vi "Dashboard Main.vi"() -> ()   [LabVIEW 2019]
uses:
  <vilib>/Utility/miscctls.llb/LVRowAndColumnTypeDef.ctl
  <vilib>/event_ctls.llb/eventvkey.ctl
  <vilib>/Rock Robotics/Network Tables/NT Write Boolean.vi
  <vilib>/Utility/file.llb/Read Delimited Spreadsheet (string).vi
  <vilib>/Rock Robotics/Network Tables/NT Write String Array.vi
  <vilib>/Rock Robotics/WPI/Dashboard/WPI_DashboardLogging Global.vi
panel:
  in  "Camera Settings Right":T1={"Frame Rate"=30, "Compression"=30, "Size"=1, "DB Camera Config"=FALSE} {"Frame Rate" scale=1.0..30.0; "Compression" scale=100.0..-1.0; "Size" items=["640x480", "320x240", "160x120"]}
  in  "Camera Name Right":string(combo)="No Camera Selection"
  out "Camera Perf":string
  in  "Camera Settings":T1={"Frame Rate"=30, "Compression"=30, "Size"=1, "DB Camera Config"=FALSE} {"Frame Rate" scale=1.0..30.0; "Compression" scale=100.0..-1.0; "Size" items=["640x480", "320x240", "160x120"]}
  in  "TCP":refnum<k5>
  in  "Rec Mode":enum32{"Stop", "Record", "Playback"}(radio)
  out "Robot IP":string
  out "Image Message":string="Timeout in Camera Communications"
  in  "Dashboard Tab":T2(tab)
  in  "Select Auto":string(combo)="Select Autonomous ..."
  out "NT Connection":bool
  out "JS1 Z":dbl(slide) scale=-1.0..1.0 scale format="%#_2e"
  out "JS1 Graph":cluster{"X":dbl, "Y":dbl}[](graph)
  out "JS1 Buttons":T3
  out "JS2 Z":dbl(slide) scale=-1.0..1.0 scale format="%#_2e"
  out "JS2 Graph":cluster{"X":dbl, "Y":dbl}[](graph)
  out "JS2 Buttons":T3
  out "Mode":T4(ring)=enum."Auto Disabled"
  out "Right Camera Perf":cluster{"Bandwidth (Mbps)":dbl, "FPS":dbl}
  out "Camera Image Right":T5(plugin-control)
  in  "DB/String 9":string
  in  "DB/String 8":string
  in  "DB/String 7":string
  in  "DB/String 6":string
  in  "DB/String 5":string
  in  "DB/String 4":string
  in  "DB/String 3":string
  in  "DB/String 2":string
  in  "DB/String 1":string
  in  "DB/String 0":string
  in  "DB/Slider 0":dbl(slide) scale=0.0..5.0
  in  "DB/Slider 1":dbl(slide) scale=0.0..5.0
  in  "DB/Slider 2":dbl(slide) scale=0.0..5.0
  in  "DB/Slider 3":dbl(slide) scale=0.0..5.0
  out "DB/LED 3":bool
  out "DB/LED 2":bool
  out "DB/LED 1":bool
  out "DB/LED 0":bool
  in  "DB/Button 3":bool
  in  "DB/Button 2":bool
  in  "DB/Button 1":bool
  in  "DB/Button 0":bool caption="New Name"
  in  "Test Slider":dbl(slide) scale=0.0..100.0 scale format="%#_3g"
  in  "On/Off":bool caption="Solenoid"
  in  "Test Name":u16(ring) items=["Select the test to run..."]
  in  "Test Tree":string(tree)
  in  "Motor":cluster{"Value":dbl, "Enable":bool} {"Value" scale=-1.0..1.0 scale format="%#_3g"}
  out "Progress":T6 {"Test Progress" scale=0.0..100.0}
  in  "Rev/Fwd":cluster{"Forward":bool, "Reverse":bool}
  in  "Test Ring":u16(ring) items=["Monochrome", "Color"]
  out "Cmd Status":string
  in  "Execute Command":bool
  in  "Command Params":string[][](table)
  in  "Command Selection":i32(listbox)
  in  "CheckList":i32(listbox)
  out "Tree":string(tree)
  out "Magazine":enum32{"Controls", "Indicators"}(tab)
  in  "Max Magazine Speed":dbl
  in  "Unjam Speed":dbl
  in  "Firing Speed":dbl
  in  "Loading Speed":dbl
  in  "Bottom IR Theshold":dbl
  in  "Bottom Middle IR Threshold":dbl
  in  "Top Middle IR Threshold":dbl
  in  "Top IR Threshold":dbl
  out "Current Max Magazine Speed":dbl
  out "Current Unjam Speed":dbl
  out "Current Firing Speed":dbl
  out "Current Loading Speed":dbl
  out "Current Bottom IR Threshold":dbl
  out "Current Bottom Middle IR Threshold":dbl
  out "Current Top Middle IR Threshold":dbl
  out "Current Top IR Threshold":dbl
  in  "Boolean":bool
  out "Drive":enum32{"Controls", "Indicators"}(tab)
  in  "Left P":dbl
  in  "Left I":dbl
  in  "Left D":dbl
  in  "Left F":dbl
  in  "Right P":dbl
  in  "Right I":dbl
  in  "Right D":dbl
  in  "Right F":dbl
  out "Current Right F":dbl
  out "Current Right D":dbl
  out "Current Right I":dbl
  out "Current Right P":dbl
  out "Current Left F":dbl
  out "Current Left D":dbl
  out "Current Left I":dbl
  out "Current Left P":dbl
  out "Flywheel":enum32{"Controls", "Indicators"}(tab)
  in  "Flywheel Max":dbl
  in  "Flywheel Min":dbl
  in  "Flywheel I":dbl
  in  "Flywheel F":dbl
  in  "Flywheel D":dbl
  in  "Flywheel I":dbl
  in  "Flywheel P":dbl
  out "Current Flywheel Max":dbl
  out "Current Flywheel Min":dbl
  out "Current Flywheel I":dbl
  out "Current Flywheel F":dbl
  out "Current Flywheel D":dbl
  out "Current Flywheel I":dbl
  out "Current Flywheel P":dbl
  out "Turret":enum32{"Controls", "Indicators"}(tab)
  in  "Turret Upper Limit":dbl
  in  "Turret Lower Limit":dbl
  out "Current Turret Lower Limit":dbl
  out "Current Turret Upper Limit":dbl
  out "Climb":enum32{"Controls", "Indicators"}(tab)
  in  "Climb I":dbl
  in  "Climb P":dbl
  in  "Climb D":dbl
  out "Current Climb D":dbl
  out "Current Climb I":dbl
  out "Current Climb P":dbl
  out "Intake":enum32{"Controls", "Indicators"}(tab)
  in  "extend delay(ms)":dbl
  in  "retract delay(ms)":dbl
  in  "Intake Speed":dbl
  out "Current Intake Speed":dbl
  out "Current Magazine Speed":dbl
  out "Match Color":string
  in  "Auto Selector":u16(ring) items=["Trench Play", "Move Off Line", "No Auto"]
  out "Camera Image":T5(plugin-control)
  out "Background":bool
  in  "Camera Name":string(combo)="No Camera Selection"
  # "HW"
  # "HW"
  # "Joysticks"
  # "Drive Motors"
  # "Front"
  # "Right"
  # "Left"
  # "Back"
  # "This tab is a great place for autonomous settings and robot-specific values.\nPlace controls and indicators inside this tab and match name to\nDashboard Variables on robot. You can also delete this comment."
  # "Read"
  # "Write"
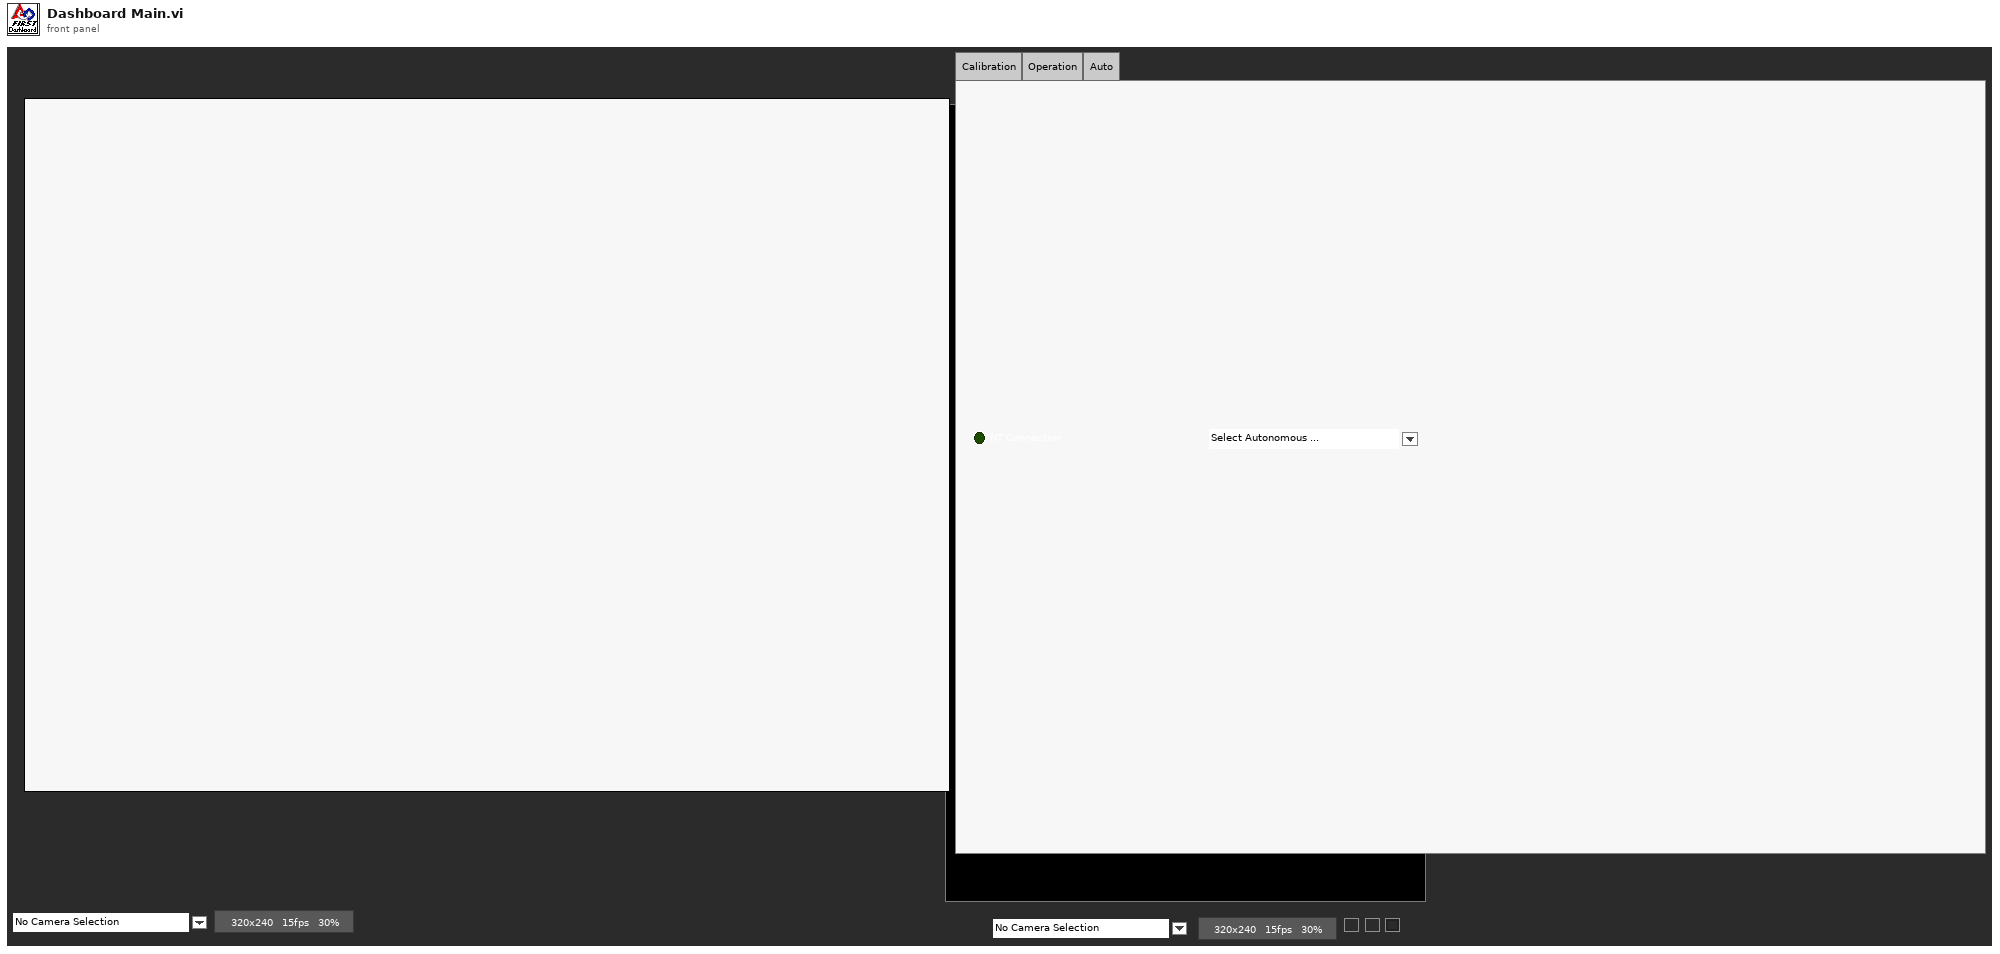
[diagram p1: front panel]
types:
  T1 = cluster{"Frame Rate":i32, "Compression":i32, "Size":u16, "DB Camera Config":bool}
  T2 = enum32{"Drive", "Camera", "Basic", "Custom", "Test", "Commands", "Checklist", "Variables", "Calibration", "Operation", "Auto"}
  T3 = cluster{bool, bool, bool, bool, bool, bool, bool, bool, bool, bool, bool, bool}
  T4 = enum8{"Tele-Op Disabled", "Tele-Op Enabled", "Auto Disabled", "Auto Enabled", "Test Disabled", "Test Enabled", "Disconnected", "No Code", "E-Stop"}
  T5 = typedef "IMAQ Image.ctl" = refnum<image>
  T6 = cluster{"Test Progress":u8, "Test Progress Text":string}
  T7 = cluster{"Save Path":path, "Interval (s)":dbl, "Keep":i32}
  T8 = enum32{"Drive", "Camera", "Basic", "Custom", "Test", "Commands", "Checklist", "Variables"}
  T9 = typedef "Image Type" = u32
  T10 = cluster{"IDs":cluster{"RPC field ID":u16, "Unique ID":u16}, "String":string}
  T11 = cluster{"Error Strings":string, "Disable Counts":cluster{u16, u16}, "Rail Faults":cluster{u16, u16, u16}, "Robot IP":string, "DB Mode":u8, "Event Info":cluster{"Name":string, "Type":u8, "Number":u16, "Replay":u8}}
  T12 = cluster{"Storage":cluster{"Disk Free":u64, "RAM Block":u32, "RAM free":u32}, "CPU Utilization":cluster{"CPU % ISR":sgl, "CPU % Time Crit":sgl, "CPU % Timed Str":sgl, "CPU % High":sgl, "CPU % Above":sgl, "CPU % Normal":sgl, "CPU % Low":sgl}, "CAN":cluster{"% Bus Utilization":sgl, "Bus Off Cnt":u32, "TX_FIFO Full Cnt":u32, "Receive Error Cnt":u8, "Transmit Error Cnt":u8}, "HID":cluster{"HID Outputs":u32, "Rumble Low":u16, "Rumble High":u16}[]}
  T13 = cluster{"Status bits":cluster{"Test Mode":bool, "Autonomous":bool, "Enabled":bool, "Code Start":bool, "Brownout":bool, "Reserved 2":bool, "Reserved 3":bool, "E-Stop":bool}, "Code Trace":cluster{"Disabled":bool, "TeleOp":bool, "Auto":bool, "Test":bool}, "Controller Type":enum16{"unknown", "cRIO", "roboRio"}, "Code?":enum16{"unknown", "noCode", "code"}, "Battery V":dbl}
  T14 = cluster{"Control Bits":cluster{"TestMode":bool, "Autonomous":bool, "Enabled":bool, "FMS Present":bool, bool, bool, bool, "E-Stop":bool}, "Team Station ":u8, "Countdown":sgl, "Joystick Values":cluster{"Axes":dbl[], "Buttons":bool[], "POVs":i16[]}[]}
  T15 = cluster{"Axes":dbl[], "Buttons":bool[], "POVs":i16[]}[]
  T16 = cluster{"Axes":dbl[], "Buttons":bool[], "POVs":i16[]}
  T17 = cluster{"Buttons[0]":bool, "Buttons[1]":bool, "Buttons[2]":bool, "Buttons[3]":bool, "Buttons[4]":bool, "Buttons[5]":bool, "Buttons[6]":bool, "Buttons[7]":bool, "Buttons[8]":bool, "Buttons[9]":bool, "Buttons[10]":bool, "Buttons[11]":bool}
  T18 = cluster{"Camera Image":refnum<vi>, "Dashboard Tab":refnum<vi>, "Background":refnum<vi>, "Rec Mode":refnum<vi>, "Test Slider":refnum<vi>, "On/Off ":refnum<vi>, "Test Ring":refnum<vi>, "Rev/Fwd":refnum<vi>, "Test Name":refnum<vi>, "Motor":refnum<vi>, "Progress":refnum<vi>, "CheckList":refnum<vi>, "Tree":refnum<vi>, "Test Tree":refnum<vi>, "Command Params":refnum<vi>, "Command Selection":refnum<vi>, "Execute Command":refnum<vi>, "Cmd Status":refnum<vi>, "Camera Settings":refnum<vi>, "Camera Name":refnum<vi>, "Camera Perf":refnum<vi>, "Camera Settings Right":refnum<vi>, "Camera Name Right":refnum<vi>, "Camera Image Right":refnum<vi>}
  T19 = cluster{"Global Rectangle":i32[], "Contours":cluster{"Contour Type":u32, "ROI Type":u32, "Points":i32[]}[]}
  T20 = cluster{"Camera Name":string, string, "Saved DB Images Info":cluster{"Save Path":path, "Interval (s)":dbl, "Keep":i32}}
  T21 = cluster{"Camera Name Right":string, string, "Saved DB Images Info":cluster{"Save Path":path, "Interval (s)":dbl, "Keep":i32}}
  T22 = cluster{"Operation":enum16{"Update", "Clear"}, "Color Box":u32}[]
  T23 = typedef "eventvkey.ctl" = enum16{"ASCII", "Enter", "Return", "Shift", "Ctrl", "Alt", "Cmd", "Opt", "Caps", "NumLock", "Clear", "Break", "Up", "Down", "Left", "Right", "Insert", "Delete", "Home", "End", "PageUp", "PageDown", "Escape", "Help", "Pause", "ScrollLock", "F1", "F2", "F3", "F4", "F5", "F6", "F7", "F8", "F9", "F10", "F11", "F12", "F13", "F14", "F15", "F16", "F17", "F18", "F19", "F20", "F21", "F22", "F23", "F24", "Play", "VolumeUp", "VolumeDown", "Mute", "Two Byte Char"}
  T24 = cluster{"Image Size":bool, "Image Type":bool, "Pixel Value":bool, "ROI Information":bool, "Zoom Factor":bool}
  T25 = cluster{"Operation":enum16{"Update", "Clear"}, "Color Box":u32}
  T26 = typedef "LVRowAndColumnTypeDef.ctl" = cluster{"Row":i32, "Column":i32}
  T27 = cluster{"Shift":bool, "Ctrl":bool, "Alt":bool, "Cmd":bool, "Opt":bool}
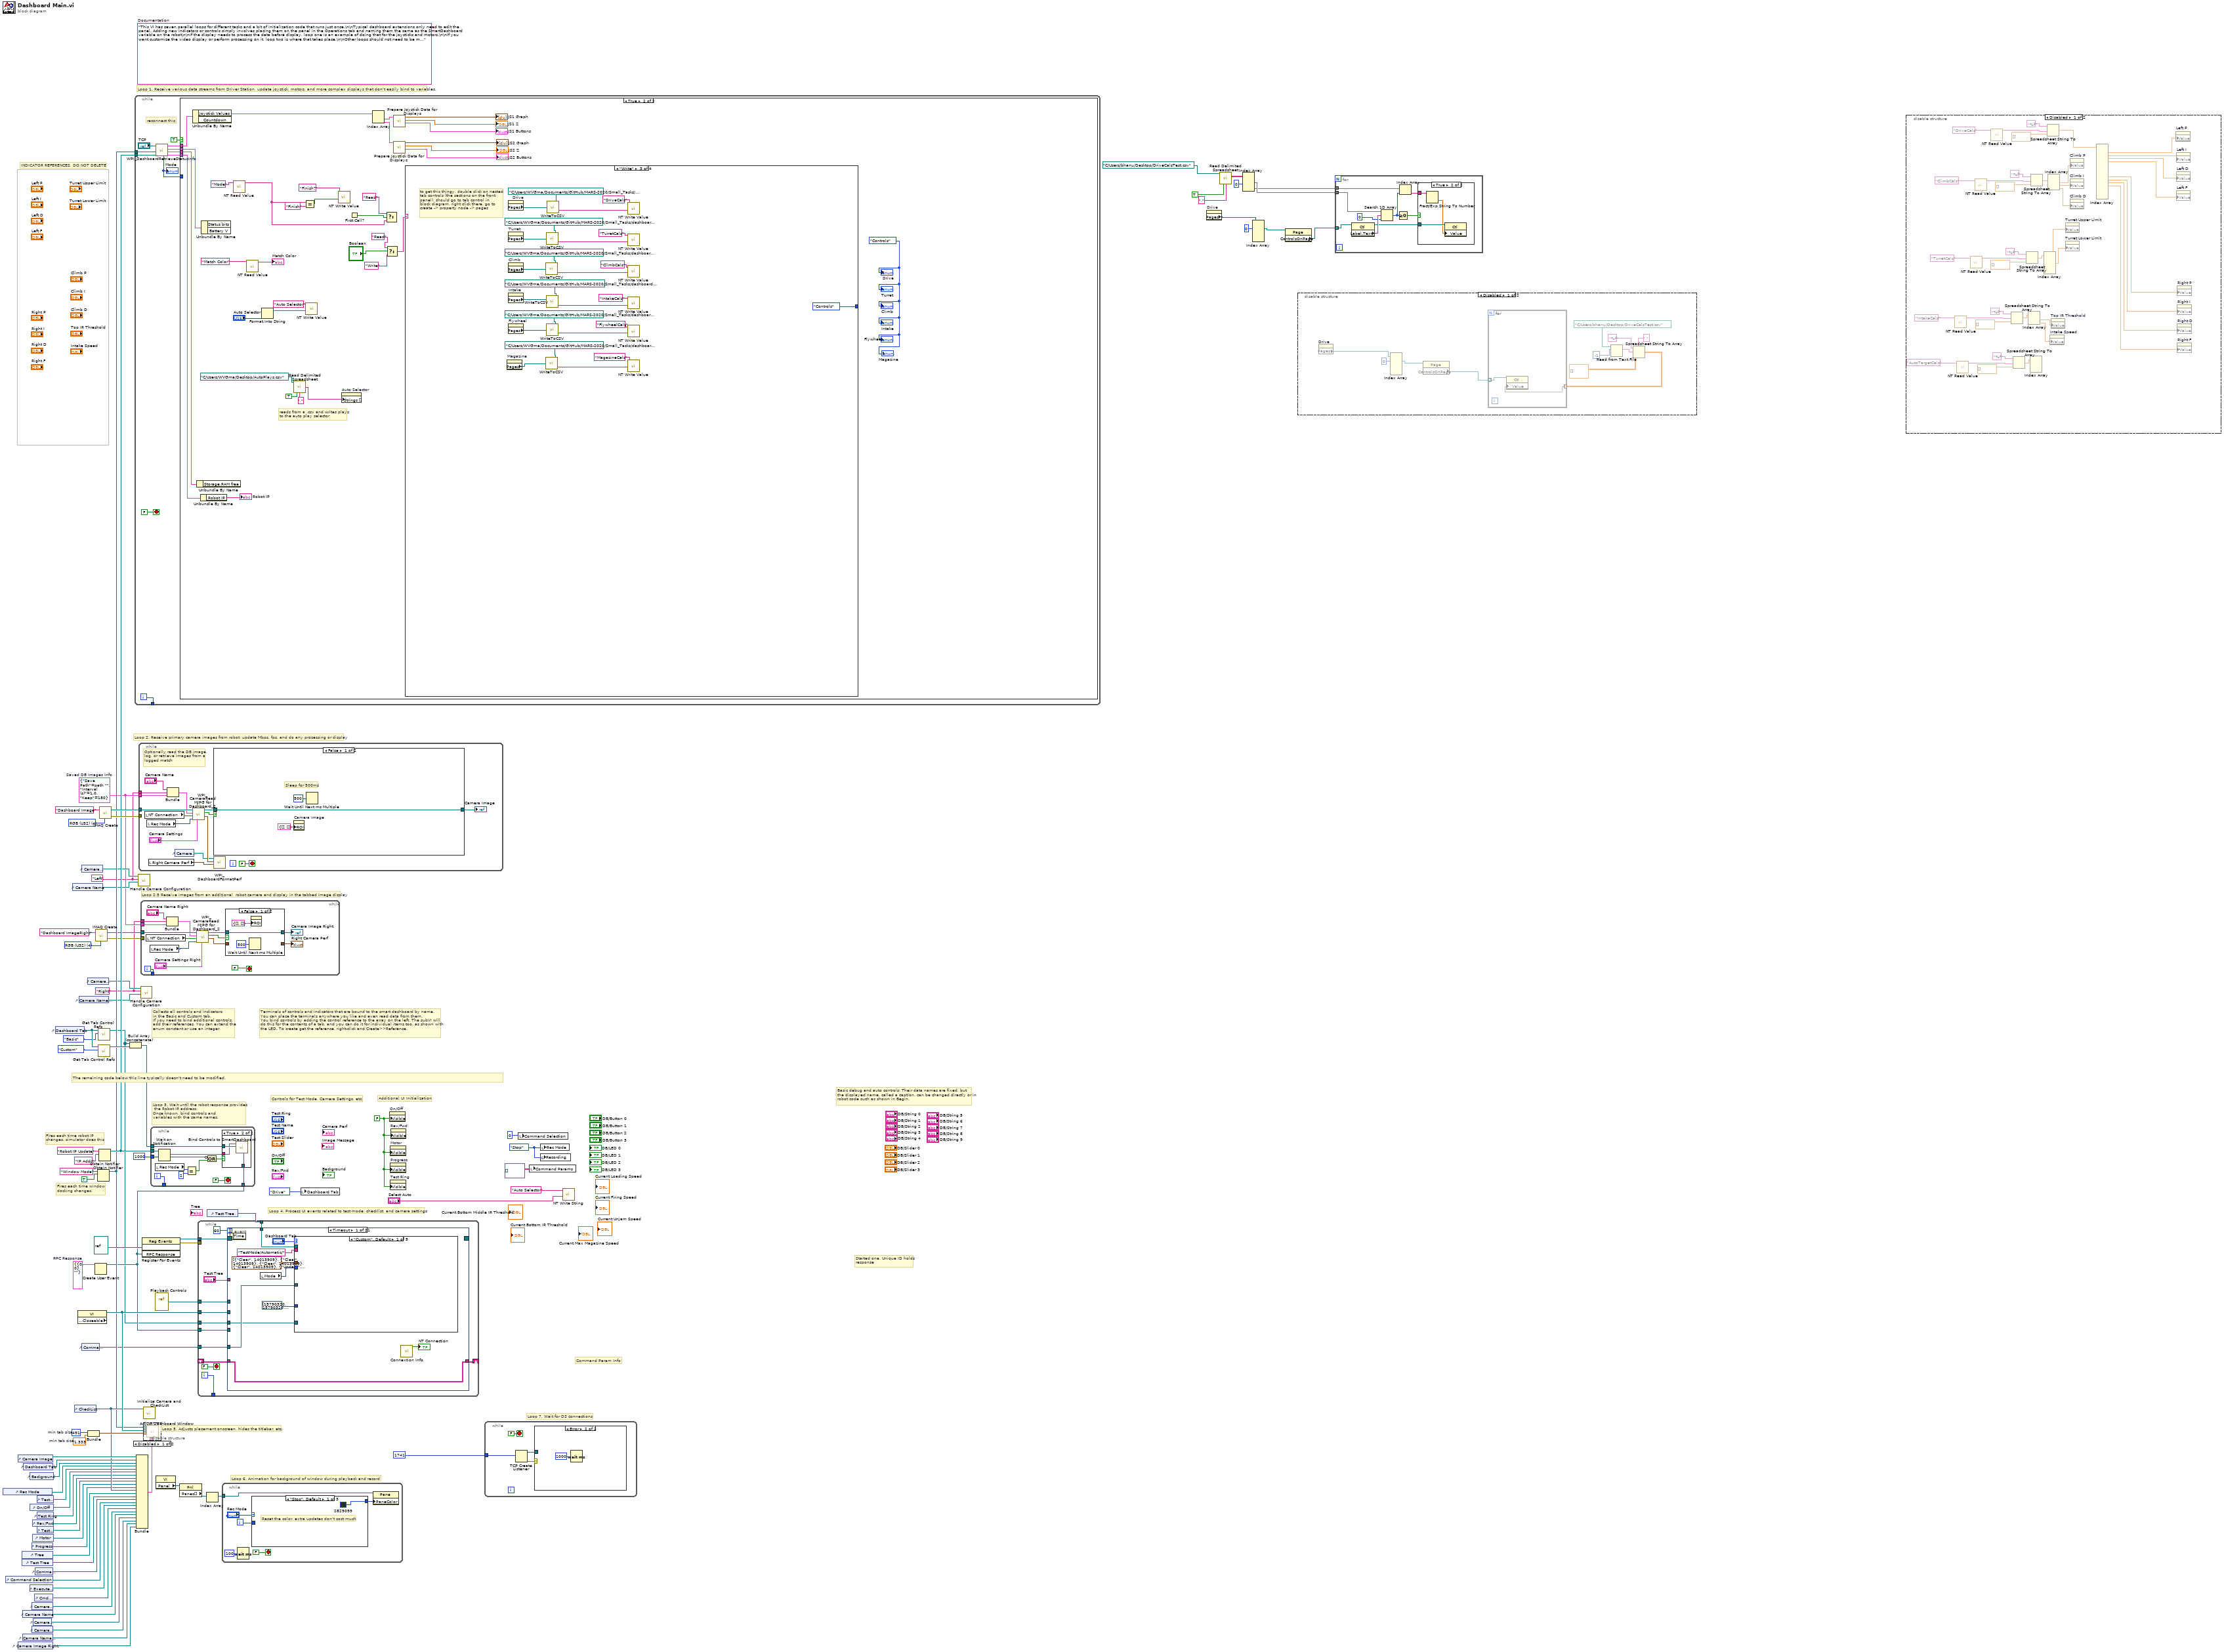
[diagram p0: block diagram]
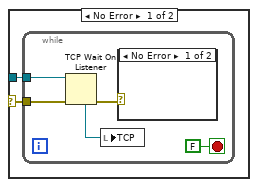
[diagram p7: hidden frame]
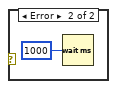
[diagram p8: hidden frame]
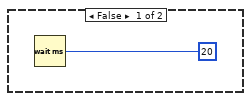
[diagram p9: hidden frame]
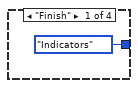
[diagram p10: hidden frame]
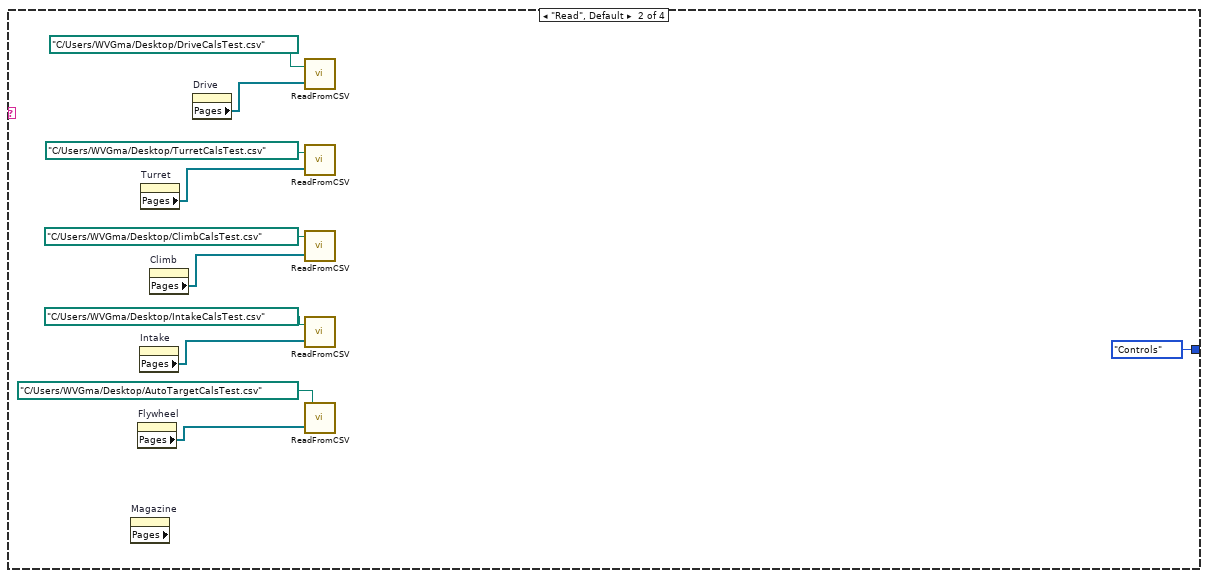
[diagram p11: hidden frame]
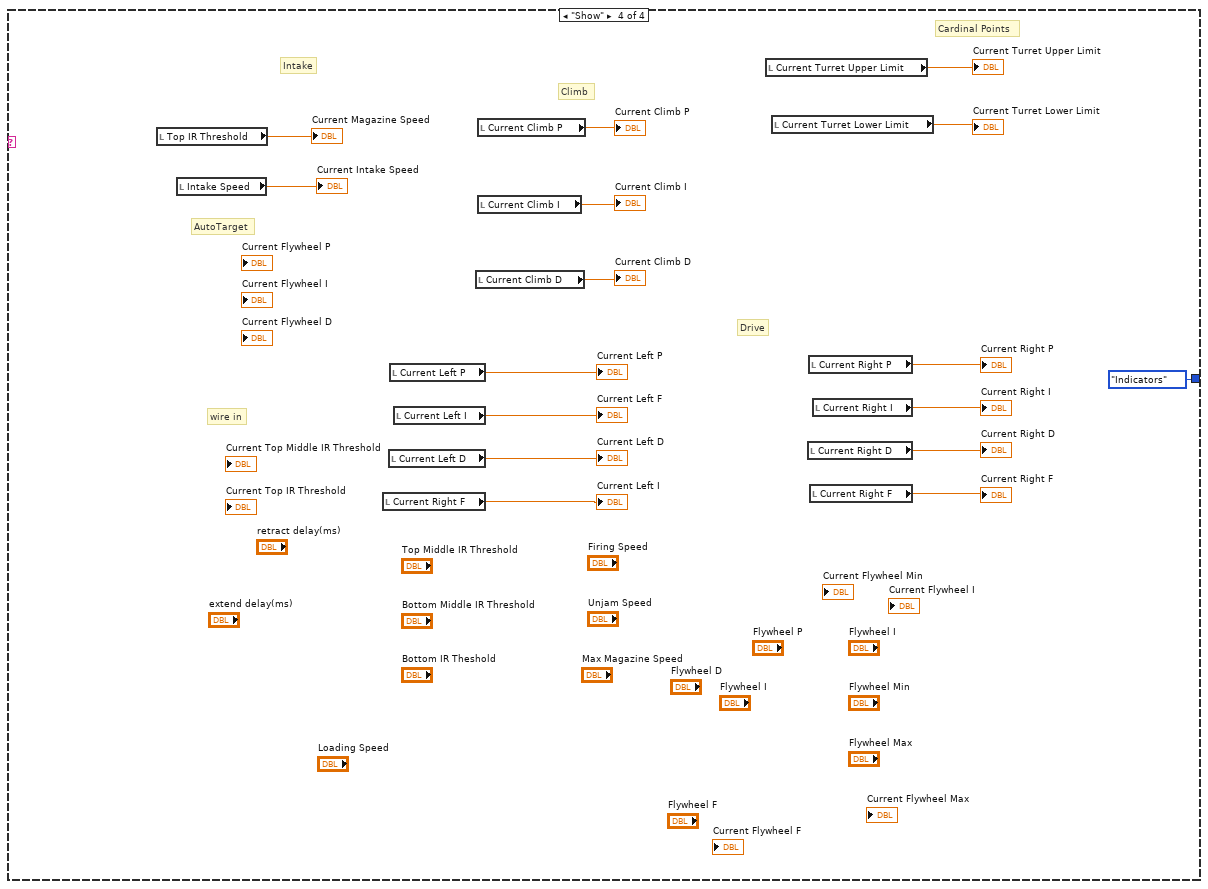
[diagram p12: hidden frame]
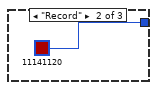
[diagram p13: hidden frame]
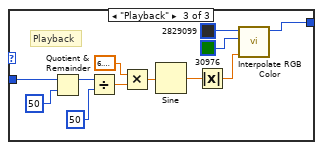
[diagram p14: hidden frame]
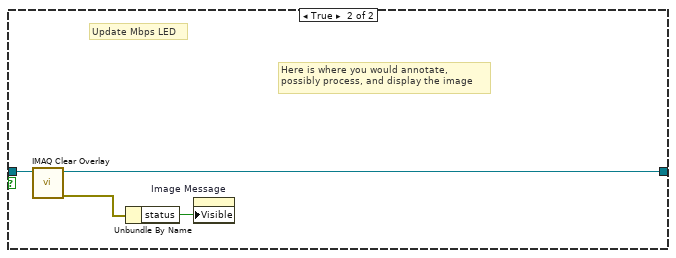
[diagram p16: hidden frame]
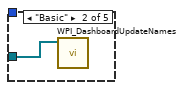
[diagram p17: hidden frame]
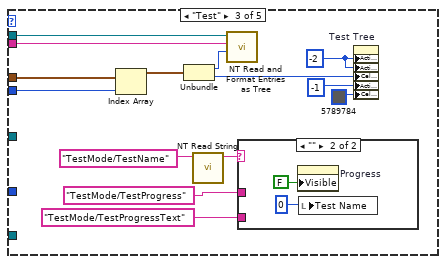
[diagram p18: hidden frame]
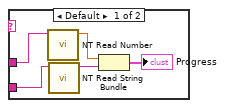
[diagram p19: hidden frame]
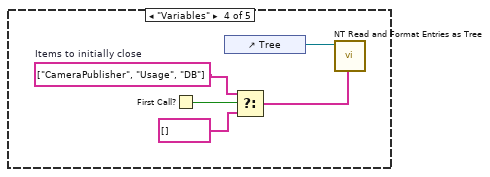
[diagram p20: hidden frame]
diagram:
  w14 = T7 {"Save Path"=path "", "Interval (s)"=1.0, "Keep"=180}  # Saved DB Images Info
  w13 = "Right"
  w12 = "Left"
  w24 = T9 4 items=["Grayscale (U8)", "Grayscale (I16)", "Grayscale (SGL)", "Complex (CSG)", "RGB (U32)", "HSL (U32)", "RGB (U64)"] ("Image Type")
  w40 = T10 {"IDs"={"RPC field ID"=0, "Unique ID"=0}, "String"=""}  # RPC Response
  w63 = 491  # min tab size
  w62 = 1.333  # min tab size
  w70 = enum32{"Stop", "Record", "Playback"}."Stop" ("Rec Mode")
  w47 = FALSE ("Visible")
  (unwired) "This VI has seven parallel loops for different tasks and a bit of initialization code that runs just once.\n\nTypical dashboard extensions only need to edit the panel. Adding new indicators or controls simply involves placing them on the panel in the Operations tab and naming them the same as the SmartDashboard variable on the robot\n\nIf the display needs to process the data before display, loop one is an example of doing that for the joysticks and motors.\n\nIf you want customize the video display or perform processing on it, loop two is where that takes place.\n\nOther loops should not need to be modified. They are pretty standard, and document the task they perform."  # Documentation
  w87 = T9 4 items=["Grayscale (U8)", "Grayscale (I16)", "Grayscale (SGL)", "Complex (CSG)", "RGB (U32)", "HSL (U32)", "RGB (U64)"] ("Image Type")
  # "INDICATOR REFERENCES, DO NOT DELETE"
  # "Loop 2.5 Receive images from an additional  robot camera and display in the tabbed image display"
  # "Command Param Info"
  # "Started one, Unique ID holds\nresponse"
  # "Loop 7. Wait for DS connections"
  # "Basic debug and auto controls: Their data names are fixed, but\nthe displayed name, called a caption, can be changed directly or in\nrobot code such as shown in Begin."
  # "Controls for Test Mode, Camera Settings, etc."
  # "Additional UI Initialization"
  # "Loop 6. Animation for background of window during playback and record"
  # "Fires each time robot IP\nchanges, simulator does this"
  # "Fires each time window\ndocking changes."
  # "Collects all controls and indicators\nin the Basic and Custom tab.\nIf you need to bind additional controls,\nadd their references. You can extend the\nenum constant or use an integer."
  # "The remaining code below this line typically doesn't need to be modified."
  # "Loop 4. Process UI events related to test mode, checklist, and camera settings"
  # "Terminals of controls and indicators that are bound to the smart dashboard by name.\nYou can place the terminals anywhere you like and even read data from them.\nYou bind controls by adding the control reference to the array on the left. The subVI will\ndo this for the contents of a tab, and you can do it for individual items too, as shown with\nthe LED. To create get the reference, right-click and Create>>Reference."
  # "Loop 3. Wait until the robot response provides\n the Robot IP address.\nOnce known, bind controls and\nvariables with the same names."
  # "Loop 5. Adjusts placement onscreen, hides the titlebar, etc."
  # "Loop 1. Receive various data streams from Driver Station, update joystick, motors, and more complex displays that don't easily bind to variables."
  # "Loop 2. Receive primary camera images from robot, update Mbps, fps, and do any processing or display"
  n1 = control-ref of="Rec Mode"() -> (w53:refnum<vi>)
  n2 = control-ref of="Command Selection"() -> (w39:refnum<vi>)
  n3 = control-ref of="Camera Image Right"() -> (w17:refnum<vi>)
  n4 = control-ref of="Camera Image"() -> (w65:refnum<vi>)
  n5 = control-ref of="Tree"() -> (w57:refnum<vi>)
  n6 = control-ref of="Test Tree"() -> (w56:refnum<vi>)
  n7 = control-ref of="Camera Name"() -> (w30:refnum<vi>)
  n8 = control-ref of="Camera Name Right"() -> (w18:refnum<vi>)
  n9 = control-ref of="Dashboard Tab"() -> (w64:refnum<vi>)
  n10 = control-ref of="Execute Command"() -> (w41:refnum<vi>)
  n11 = control-ref of="Background"() -> (w60:refnum<vi>)
  n12 = control-ref of="On/Off"() -> (w51:refnum<vi>)
  n13 = control-ref of="Progress"() -> (w48:refnum<vi>)
  n14 = control-ref of="Camera Settings"() -> (w31:refnum<vi>)
  n15 = control-ref of="Camera Settings Right"() -> (w19:refnum<vi>)
  n16 = control-ref of="Rev/Fwd"() -> (w49:refnum<vi>)
  n17 = control-ref of="Motor"() -> (w54:refnum<vi>)
  n18 = control-ref of="Camera Perf"() -> (w29:refnum<vi>)
  n19 = control-ref of="Cmd Status"() -> (w35:refnum<vi>)
  n20 = control-ref of="Command Params"() -> (w42:refnum<vi>)
  n21 = control-ref of="Test Slider"() -> (w52:refnum<vi>)
  n22 = control-ref of="Test Ring"() -> (w50:refnum<vi>)
  n23 = control-ref of="Test Name"() -> (w55:refnum<vi>)
  n24 = control-ref of="Dashboard Tab"() -> (w68:refnum<vi>)
  n25 = control-ref of="Camera Name"() -> (w32:refnum<vi>)
  n26 = control-ref of="CheckList"() -> (w58:refnum<vi>)
  n27 = property class="VI" props=["Front Panel.Closeable"]() -> (reference out=w69:refnum<vi>)  [unwired: 2 in, 2 out]
  n28 = control-ref of="Camera Name Right"() -> (w20:refnum<vi>)
  n29 = control-ref of="Camera Settings"() -> (w33:refnum<vi>)
  n30 = control-ref of="Command Params"() -> (w34:refnum<vi>)
  n31 = control-ref of="Camera Settings Right"() -> (w21:refnum<vi>)
  n32 = Bundle("min tab size"=w63, "min tab size"=w62) -> (w61:cluster{"min tab size":i32, "min tab size":dbl})  [unwired: 1 in]
  n33 = Create User Event(user event datatype=w40) -> (user event=w36:refnum<user-event>)  [unwired: 1 in, 1 out]
  n34 = call "IMAQ Create"("Image Name"="Dashboard ImageRight", "Image Type"=w24) -> ("New Image"=w23:T5, "error out"=w22:errorcluster)  [unwired: 2 in, 1 out]
  n35 = Obtain Notifier(name (unnamed)="Window Mode", notification data type=TRUE) -> (notifier out=w45:refnum<notifier>)  [unwired: 2 in, 2 out]
  n36 = call <vilib>:"Get Tab Control Refs.vi"("Page Index"=T8."Basic" ("Dashboard Tab"), "TabControl in"=w68) -> ("ControlsOnPage"=w28:refnum<vi>[])  [unwired: 9 in]
  n37 = call <vilib>:"Get Tab Control Refs.vi"("Page Index"=T8."Custom" ("Dashboard Tab"), "TabControl in"=w68) -> ("ControlsOnPage"=w67:refnum<vi>[])  [unwired: 9 in]
  n38 = Obtain Notifier(name (unnamed)="Robot IP Update", notification data type="IP Addr" ("name (unnamed)")) -> (notifier out=w46:refnum<notifier>)  [unwired: 2 in, 2 out]
  n39 = call "IMAQ Create"("Image Name"="Dashboard Image", "Image Type"=w87) -> ("New Image"=w85:T5, "error out"=w84:errorcluster)  [unwired: 2 in, 1 out]
  n40 = Build Array (concatenate)(w28, w67) -> (w66:refnum<vi>[])
  n41 = while {
    tunnel: [w97] -> _
    tunnel: w46 -> [w92]
    tunnel: w45 -> [w89]
    i -> [w97]
    stop <- FALSE stop-if-true
    # "reconnect this"
    n42 = call <vilib>:"WPI_DashboardRetrieveStatusInfo.vi"("Binding Refnum"=w92, "Window Mode Notifier"=w89, "TCP Cnx"="TCP") -> ("Power and Errors"=w93:T11, "Robot Metrics"=w95:T12, "Status Info"=w96:T13, "Control Info"=w94:T14, "Robot Mode"=w91:T4)  [unwired: 3 in, 1 out]
    "Mode" <- w91
    n43 = case shown="True" TRUE {
      tunnel: w96 -> [_ w134]
      tunnel: w95 -> [_ w133]
      tunnel: w94 -> [_ w132]
      tunnel: w93 -> [_ w131]
      tunnel: w91 -> [_ _]
      frame False {
        n44 = Wait (ms)(milliseconds to wait=u32 20) -> ()  [unwired: 1 out]
      }
      frame True {
        w100 = enum32{"Controls", "Indicators"}."Controls" ("Climb")
        # "reads from a .csv and writes plays\nto the auto play selector"
        n45 = Unbundle By Name(w132) -> ("Joystick Values"=w130:T15)  [unwired: 1 out]
        n46 = Unbundle By Name(w133) -> ()  [unwired: 1 out]
        n47 = Unbundle By Name(w131) -> ("Robot IP"=→"Robot IP":string)
        n48 = Unbundle By Name(w134) -> ()  [unwired: 2 out]
        n49 = call-poly <vilib>:"NT Read Value.vi"("Name"="Mode") -> ("String"=w114:string)  [unwired: 9 in, 1 out]
        n50 = call-poly <vilib>:"NT Read Value.vi"("Name"="Match Color") -> ("String"=→"Match Color":string)  [unwired: 9 in, 1 out]
        n51 = Format Into String("Auto Selector") -> (resulting string=w111:string)  [unwired: 3 in, 1 out]
        n52 = call-poly <vilib>:"Read Delimited Spreadsheet.vi"("file path (dialog if empty)"=path "C:/Users/WVGma/Desktop/AutoPlays.csv", "transpose? (F)"=TRUE, "delimiter (\\t)"="," ("delimiter (\\t)")) -> ("first row"=w105:string[])  [unwired: 7 in, 5 out]
        n53 = Equal?(x=w114, y="Finish") -> (x = y?=w118:bool)
        n54 = call-poly <vilib>:"NT Write Value.vi"("String"=w111, "Name"="Auto Selector") -> ()  [unwired: 9 in, 1 out]
        n55 = call-poly <vilib>:"NT Write Value.vi"("Boolean"=w118, "Name"="Finish?") -> ()  [unwired: 9 in, 1 out]
        n56 = property on="Auto Selector" class="Ring (strict)"("Strings []"=w105) -> ()  [unwired: 2 in, 2 out]
        n57 = First Call?() -> (First Call?: T/F=w116:bool)
        n58 = Index Array(array=w130) -> (element #1=w129:T16, element #2=w125:T16)  [unwired: 2 in]
        n59 = Select(t="Read" ("f"), s=w116, f=w114) -> ()  [unwired: 1 out]
        n60 = Select(t="Read", s="Boolean", f="Write") -> (s? t:f=w101:string)
        n61 = call "Prepare Joystick Data for Displays.vi"("Joystick Values"=w125) -> ("Buttons"=→"JS2 Buttons":T17, "Z Axis"=→"JS2 Z":dbl, "Cartesian Data"=→"JS2 Graph":cluster{"X axis":dbl, "X axis":dbl}[])  [unwired: 8 in]
        n62 = call "Prepare Joystick Data for Displays.vi"("Joystick Values"=w129) -> ("Buttons"=→"JS1 Buttons":T17, "Z Axis"=→"JS1 Z":dbl, "Cartesian Data"=→"JS1 Graph":cluster{"X axis":dbl, "X axis":dbl}[])  [unwired: 8 in]
        n63 = case shown="\"Write\"" w101 {
          tunnel: [enum32{"Controls", "Indicators"}."Indicators" ("Climb") enum32{"Controls", "Indicators"}."Controls" ("Climb") enum32{"Controls", "Indicators"}."Controls" ("Climb") enum32{"Controls", "Indicators"}."Indicators" ("Climb")] -> _
          frame "Finish" {
          }
          frame "Read", Default {
            n64 = property on="Magazine" class="TabCtl (strict)" props=["Pages"]() -> ()  [unwired: 2 in, 3 out]
            n65 = property on="Flywheel" class="TabCtl (strict)"() -> ("Pages"=w136:refnum<vi>[])  [unwired: 2 in, 2 out]
            n66 = property on="Intake" class="TabCtl (strict)"() -> ("Pages"=w137:refnum<vi>[])  [unwired: 2 in, 2 out]
            n67 = property on="Turret" class="TabCtl (strict)"() -> ("Pages"=w142:refnum<vi>[])  [unwired: 2 in, 2 out]
            n68 = property on="Climb" class="TabCtl (strict)"() -> ("Pages"=w138:refnum<vi>[])  [unwired: 2 in, 2 out]
            n69 = property on="Drive" class="TabCtl (strict)"() -> ("Pages"=w144:refnum<vi>[])  [unwired: 2 in, 2 out]
            n70 = call "ReadFromCSV.vi"("Pages"=w144, "file path (dialog if empty)"=path "C:/Users/WVGma/Desktop/DriveCalsTest.csv") -> ()  [unwired: 1 in]
            n71 = call "ReadFromCSV.vi"("Pages"=w142, "file path (dialog if empty)"=path "C:/Users/WVGma/Desktop/TurretCalsTest.csv") -> ()  [unwired: 1 in]
            n72 = call "ReadFromCSV.vi"("Pages"=w138, "file path (dialog if empty)"=path "C:/Users/WVGma/Desktop/ClimbCalsTest.csv") -> ()  [unwired: 1 in]
            n73 = call "ReadFromCSV.vi"("Pages"=w137, "file path (dialog if empty)"=path "C:/Users/WVGma/Desktop/IntakeCalsTest.csv") -> ()  [unwired: 1 in]
            n74 = call "ReadFromCSV.vi"("Pages"=w136, "file path (dialog if empty)"=path "C:/Users/WVGma/Desktop/AutoTargetCalsTest.csv") -> ()  [unwired: 1 in]
          }
          frame "Write" {
            # "to get this thingy, double click on nested\ntab controls (the sections on the front \npanel), should go to tab control in \nblock diagram, right click there, go to\ncreate -> property node -> pages"
            n75 = property on="Magazine" class="TabCtl (strict)"() -> ("Pages"=w160:refnum<vi>[])  [unwired: 2 in, 2 out]
            n76 = property on="Drive" class="TabCtl (strict)"() -> ("Pages"=w161:refnum<vi>[])  [unwired: 2 in, 2 out]
            n77 = property on="Turret" class="TabCtl (strict)"() -> ("Pages"=w168:refnum<vi>[])  [unwired: 2 in, 2 out]
            n78 = property on="Climb" class="TabCtl (strict)"() -> ("Pages"=w169:refnum<vi>[])  [unwired: 2 in, 2 out]
            n79 = property on="Intake" class="TabCtl (strict)"() -> ("Pages"=w170:refnum<vi>[])  [unwired: 2 in, 2 out]
            n80 = property on="Flywheel" class="TabCtl (strict)"() -> ("Pages"=w167:refnum<vi>[])  [unwired: 2 in, 2 out]
            n81 = call "WriteToCSV.vi"("Pages"=w169, "file path (dialog if empty)"=path "C:/Users/WVGma/Documents/GitHub/MARS-2020/Small_Tasks/dashboard mOS XIII/Calibration Files/ClimbCals.csv") -> ("output array for NT"=w152:string[])
            n82 = call "WriteToCSV.vi"("Pages"=w160, "file path (dialog if empty)"=path "C:/Users/WVGma/Documents/GitHub/MARS-2020/Small_Tasks/dashboard mOS XIII/Calibration Files/MagazineCals.csv") -> ("output array for NT"=w154:string[])
            n83 = call "WriteToCSV.vi"("Pages"=w168, "file path (dialog if empty)"=path "C:/Users/WVGma/Documents/GitHub/MARS-2020/Small_Tasks/dashboard mOS XIII/Calibration Files/TurretCals.csv") -> ("output array for NT"=w157:string[])
            n84 = call "WriteToCSV.vi"("Pages"=w167, "file path (dialog if empty)"=path "C:/Users/WVGma/Documents/GitHub/MARS-2020/Small_Tasks/dashboard mOS XIII/Calibration Files/FlywheelCals.csv") -> ("output array for NT"=w155:string[])
            n85 = call "WriteToCSV.vi"("Pages"=w170, "file path (dialog if empty)"=path "C:/Users/WVGma/Documents/GitHub/MARS-2020/Small_Tasks/dashboard mOS XIII/Calibration Files/IntakeCals.csv") -> ("output array for NT"=w156:string[])
            n86 = call "WriteToCSV.vi"("Pages"=w161, "file path (dialog if empty)"=path "C:/Users/WVGma/Documents/GitHub/MARS-2020/Small_Tasks/dashboard mOS XIII/Calibration Files/DriveCals.csv") -> ("output array for NT"=w158:string[])
            n87 = call-poly <vilib>:"NT Write Value.vi"("String Array"=w158, "Name"="DriveCals") -> ()  [unwired: 9 in, 1 out]
            n88 = call-poly <vilib>:"NT Write Value.vi"("String Array"=w157, "Name"="TurretCals") -> ()  [unwired: 9 in, 1 out]
            n89 = call-poly <vilib>:"NT Write Value.vi"("String Array"=w152, "Name"="ClimbCals") -> ()  [unwired: 9 in, 1 out]
            n90 = call-poly <vilib>:"NT Write Value.vi"("String Array"=w156, "Name"="IntakeCals") -> ()  [unwired: 9 in, 1 out]
            n91 = call-poly <vilib>:"NT Write Value.vi"("String Array"=w155, "Name"="FlywheelCals") -> ()  [unwired: 9 in, 1 out]
            n92 = call-poly <vilib>:"NT Write Value.vi"("String Array"=w154, "Name"="MagazineCals") -> ()  [unwired: 9 in, 1 out]
          }
          frame "Show" {
            # "wire in"
            # "AutoTarget"
            # "Intake"
            # "Climb"
            # "Cardinal Points"
            # "Drive"
            n93 = local read "Top IR Threshold"() -> (→"Current Magazine Speed":dbl)
            n94 = local read "Intake Speed"() -> (→"Current Intake Speed":dbl)
            n95 = local read "Current Right F"() -> (→"Current Left I":dbl)
            n96 = local read "Current Left D"() -> (→"Current Left D":dbl)
            n97 = local read "Current Left P"() -> (→"Current Left P":dbl)
            n98 = local read "Current Left I"() -> (→"Current Left F":dbl)
            n99 = local read "Current Climb D"() -> (→"Current Climb D":dbl)
            n100 = local read "Current Climb P"() -> (→"Current Climb P":dbl)
            n101 = local read "Current Climb I"() -> (→"Current Climb I":dbl)
            n102 = local read "Current Turret Upper Limit"() -> (→"Current Turret Upper Limit":dbl)
            n103 = local read "Current Turret Lower Limit"() -> (→"Current Turret Lower Limit":dbl)
            n104 = local read "Current Right D"() -> (→"Current Right D":dbl)
            n105 = local read "Current Right P"() -> (→"Current Right P":dbl)
            n106 = local read "Current Right F"() -> (→"Current Right F":dbl)
            n107 = local read "Current Right I"() -> (→"Current Right I":dbl)
          }
        }
        "Drive" <- w100
        "Turret" <- w100
        "Climb" <- w100
        "Flywheel" <- w100
        "Intake" <- w100
        "Magazine" <- w100
      }
    }
  }
  n108 = Bundle("Camera Image"=w65, "Dashboard Tab"=w64, "Background"=w60, "Rec Mode"=w53, "Test Slider"=w52, "On/Off"=w51, "Test Ring"=w50, "Rev/Fwd"=w49, "Test Name"=w55, "Motor"=w54, "Progress"=w48, "CheckList"=w58, "Tree"=w57, "Test Tree"=w56, "Command Params"=w42, "Command Selection"=w39, "Execute Command"=w41, "Cmd Status"=w35, "Camera Settings"=w31, "Camera Name"=w30, "Camera Perf"=w29, "Camera Settings Right"=w19, "Camera Name Right"=w18, "Camera Image Right"=w17) -> (w59:T18)  [unwired: 1 in]
  n109 = call "Handle Camera Configuration.vi"("CameraNameRef"=w32, "Display Name"=w12, "ClusterRef"=w33) -> ()  [unwired: 9 in]
  n110 = while {
    tunnel: w85 -> [w201]
    tunnel: w84 -> [_]
    tunnel: w14 -> [w194]
    tunnel: w12 -> [w191]
    stop <- FALSE stop-if-true
    # "Optionally read the DB image,\nlog, or retrieve images from a\nlogged match"
    n111 = local read "NT Connection"() -> (w195:bool)
    n112 = local read "Rec Mode"() -> (w198:enum32{"Stop", "Record", "Playback"})
    n113 = local read "Right Camera Perf"() -> (w189:cluster{"Bandwidth (Mbps)":dbl, "FPS":dbl})
    n114 = Bundle("Camera Name"="Camera Name", w191, "Saved DB Images Info"=w194) -> (w193:T20)  [unwired: 1 in]
    n115 = control-ref of="Camera Perf"() -> (w188:refnum<vi>)
    n116 = call <vilib>:"WPI_CameraRead MJPG for Dashboard_2.vi"("Camera Settings"="Camera Settings", "Rec Mode"=w198, "NT Connection"=w195, "Capture Info"=w193, "Image in"=w201) -> ("perf info"=w190:cluster{"Bandwidth (Mbps)":dbl, "fps":dbl}, "Active"=w199:bool, "Image\\ out"=w200:T5)  [unwired: 4 in]
    n117 = case shown="False" w199 {
      tunnel: w200 -> [w204 w207]
      tunnel: [w204 w206] -> w196
      frame False {
        # "Sleep for 500ms"
        n118 = property on="Camera Image" class="ImageControl"("ROI"=T19 {"Global Rectangle"=[], "Contours"=[]}) -> ()  [unwired: 2 in, 2 out]
        n119 = Wait Until Next ms Multiple(millisecond multiple=u32 500) -> ()  [unwired: 1 out]
      }
      frame True {
        # "Here is where you would annotate,\npossibly process, and display the image"
        # "Update Mbps LED"
        n120 = call "IMAQ Clear Overlay"("Image"=w207) -> ("error out"=w208:errorcluster, "Image Out"=w206:T5)  [unwired: 2 in, 7 out]
        n121 = Unbundle By Name(w208) -> ("status"=w209:bool)
        n122 = property on="Image Message" class="Str"("Visible"=w209) -> ()  [unwired: 2 in, 2 out]
      }
    }
    "Camera Image" <- w196
    n123 = call <vilib>:"WPI_DashboardFormatPerf.vi"("Right Camera Perf"=w189, "Performance"=w190, "String in"=w188) -> ()  [unwired: 9 in]
  }
  n124 = call "Handle Camera Configuration.vi"("CameraNameRef"=w20, "Display Name"=w13, "ClusterRef"=w21) -> ()  [unwired: 9 in]
  n125 = while {
    tunnel: w23 -> [w224]
    tunnel: w22 -> [_]
    tunnel: [w219] -> _
    tunnel: w14 -> [w215]
    tunnel: w13 -> [w212]
    i -> [w219]
    stop <- FALSE stop-if-true
    n126 = local read "NT Connection"() -> (w216:bool)
    n127 = local read "Rec Mode"() -> (w223:enum32{"Stop", "Record", "Playback"})
    n128 = Bundle("Camera Name Right"="Camera Name Right", w212, "Saved DB Images Info"=w215) -> (w214:T21)  [unwired: 1 in]
    n129 = call <vilib>:"WPI_CameraRead MJPG for Dashboard_2.vi"("Camera Settings"="Camera Settings Right", "Rec Mode"=w223, "NT Connection"=w216, "Capture Info"=w214, "Image in"=w224) -> ("perf info"=w210:cluster{"Bandwidth (Mbps)":dbl, "fps":dbl}, "Active"=w218:bool, "Image\\ out"=w221:T5)  [unwired: 4 in]
    n130 = case shown="False" w218 {
      tunnel: w221 -> [w226 w229]
      tunnel: [w226 w229] -> w217
      tunnel: [_ w228] -> w211
      tunnel: w210 -> [_ w228]
      frame False {
        n131 = Wait Until Next ms Multiple(millisecond multiple=u32 500) -> ()  [unwired: 1 out]
        n132 = property on="Camera Image Right" class="ImageControl"("ROI"=T19 {"Global Rectangle"=[], "Contours"=[]}) -> ()  [unwired: 2 in, 2 out]
      }
      frame True {
      }
    }
    "Camera Image Right" <- w217
    "Right Camera Perf" <- w211
  }
  n133 = register-events(refnum<vi> refnum, w36) -> (reference out=w74:refnum<event-registration>, error out=w73:errorcluster)  [unwired: 2 in]
  n134 = call "Initialize Camera and CheckList.vi"("ListBox in"=w58) -> ()  [unwired: 11 in]
  n135 = disable-structure shown="Disabled" {
    disable-tunnel: w69 -> [w233 _]
    disable-tunnel: w61 -> [w232 _]
    disable-tunnel: w59 -> [w231 _]
    disable-tunnel: w45 -> [w230 _]
    frame Disabled {
      n136 = call "Adjust Dashboard Window.vi"("Sizing Refnums"=w231, "Size Constraints"=w232, "VI"=w233, "WIn Mode"=w230) -> ()  [unwired: 8 in]
    }
    frame Enabled {
    }
  }
  n137 = while {
    tunnel: w66 -> [w245]
    tunnel: w46 -> [w243]
    tunnel: [w241] -> _
    tunnel: u32 1000 ("milliseconds to wait") -> [w240]
    tunnel: w36 -> [w234]
    i -> [w241]
    stop <- FALSE stop-if-true
    n138 = local read "Rec Mode"() -> (w236:enum32{"Stop", "Record", "Playback"})
    n139 = Wait on Notification(notifier=w243, timeout in ms (-1)=w240) -> (notification=w242:string, timed out?=w238:bool)  [unwired: 2 in, 2 out]
    n140 = Equal?(x=w236, y=u16 2 ("Rec Mode")) -> (x = y?=w237:bool)
    n141 = Compound Arithmetic op=OR(invert w238, w237) -> (w239:bool)
    n142 = case shown="True" w239 {
      tunnel: w245 -> [_ w248]
      tunnel: w242 -> [_ w247]
      tunnel: w234 -> [_ w246]
      frame False {
      }
      frame True {
        n143 = call <vilib>:"Bind Controls to SmartDashboard.vi"("RPC ref"=w246, "Bound Control Refs"=w248, "Server IP Address"=w247) -> ()  [unwired: 9 in]
      }
    }
  }
  n144 = vi-ref "Playback Controls.vi"() -> (w75:refnum<vi>)
  n145 = property class="VI"() -> ("Panel"=w77:refnum<vi>)  [unwired: 2 in, 2 out]
  n146 = property class="Pnl"(reference=w77) -> ("Panes[]"=w78:refnum<vi>[])  [unwired: 1 in, 2 out]
  n147 = Index Array(array=w78) -> (element=w76:refnum<vi>)  [unwired: 1 in]
  n148 = control-ref of="Test Tree"() -> (w79:refnum<vi>)
  n149 = while {
    tunnel: [w258] -> _
    tunnel: w79 -> [w257]
    tunnel: w75 -> [w256]
    tunnel: w74 -> [w255]
    tunnel: w73 -> [_]
    tunnel: w69 -> [w254]
    tunnel: w36 -> [w253]
    tunnel: w34 -> [w252]
    shift-right: [w251] -> _
    shift-left: _ -> [w250]
    tunnel: w28 -> [w249]
    i -> [w258]
    stop <- FALSE stop-if-true
    n150 = event shown="[0] Timeout" {
      selector: w255 -> [_ _ _ _ _ _ _ _ _ _ _ _ _ _ _ _ _ _ _ _ _]
      dyn-events: [_ _ _ _ _ _ _ _ _ _ _ _ _ _ _ _ w518 _ _ _ _] -> _
      timeout: u32 60 ("milliseconds to wait") -> [_ _ _ _ _ _ _ _ _ _ _ _ _ _ _ _ _ _ _ _ _]
      tunnel: w257 -> [w270 _ _ _ _ _ _ _ _ _ _ _ _ _ _ _ _ _ _ _ _]
      tunnel: "Test Tree" -> [_ _ _ _ _ _ _ _ _ _ _ w485 w493 w495 w499 w507 _ _ _ _ _]
      tunnel: w256 -> [_ _ _ _ _ _ _ _ _ _ _ _ _ _ _ _ w520 _ w538 _ _]
      tunnel: w254 -> [_ _ _ _ _ _ _ _ _ _ _ _ _ _ _ _ w516 _ _ _ _]
      tunnel: w253 -> [_ _ _ _ _ _ _ _ _ _ _ _ _ _ _ _ w514 _ _ _ _]
      tunnel: w252 -> [w265 _ _ _ _ _ w436 _ _ _ _ _ _ _ _ _ _ _ _ _ _]
      tunnel: [w264 w313 w415 w420 w429 w433 w434 w443 w453 w460 w472 w484 w491 w494 w498 w506 w513 w533 w535 w539 w552] -> w251
      tunnel: w250 -> [w264 w313 w415 w420 w429 w433 w434 _ _ w460 w472 w484 w491 w494 w498 w506 w513 w533 w535 w539 w552]
      tunnel: w249 -> [w262 _ _ _ _ _ _ _ _ _ _ _ _ _ _ _ _ _ _ _ _]
      event Timeout {
        n151 = event-data() -> ()  [unwired: 1 in, 1 out]
        n152 = local read "Mode"() -> (w267:T4)
        n153 = case shown="\"Custom\", Default" "Dashboard Tab" {
          tunnel: w270 -> [_ _ w286 _ _]
          tunnel: "TestMode/Automatic/" ("Name Pattern") -> [_ _ w285 _ _]
          tunnel: T22 [{"Operation"=enum."Clear", "Color Box"=14013909}, {"Operation"=enum."Clear", "Color Box"=14013909}, {"Operation"=enum."Clear", "Color Box"=14013909}, {"Operation"=enum."Clear", "Color Box"=14013909}, {"Operation"=enum."Update", "Color Box"=14013909}, {"Operation"=enum."Update", "Color Box"=16777215}, {"Operation"=enum."Clear", "Color Box"=14013909}, {"Operation"=enum."Clear", "Color Box"=14013909}, {"Operation"=enum."Clear", "Color Box"=14013909}] -> [_ _ w278 _ w306]
          tunnel: w267 -> [_ _ w277 _ w305]
          tunnel: u32[] [15790320, 15790320, 15790320, 15790320, 16777215, 16777215, 15790320, 15790320, 15790320] -> [_ _ _ _ w311]
          tunnel: w265 -> [_ _ _ _ w299]
          tunnel: w262 -> [_ w272 _ _ _]
          frame "Custom", Default {
          }
          frame "Basic" {
            n154 = call <vilib>:"WPI_DashboardUpdateNames.vi"("Controls on Tab"=w272) -> ()  [unwired: 11 in]
          }
          frame "Test" {
            w284 = -2 ("Active Item:Row Number")
            n155 = Index Array(array=w278, index=w277) -> (element=w279:T25)
            n156 = Unbundle(w279) -> ("Operation"=w280:enum16{"Update", "Clear"}, "Color Box"=w281:u32)
            n157 = call <vilib>:"NT Read String.vi"("Name"="TestMode/TestName") -> ("String"=w275:string)  [unwired: 9 in, 1 out]
            n158 = call <vilib>:"NT Read and Format Entries as Tree.vi"("Operation"=w280, "Name Pattern"=w285, "Tree Refnum"=w286) -> ()  [unwired: 7 in, 2 out]
            n159 = case shown="\"\"" w275 {
              tunnel: "TestMode/TestProgress" ("Name") -> [w288 _]
              tunnel: "TestMode/TestProgressText" ("Name") -> [w287 _]
              frame Default {
                n160 = call <vilib>:"NT Read Number.vi"("Name"=w288) -> ("Numeric"=w289:dbl)  [unwired: 9 in, 1 out]
                n161 = call <vilib>:"NT Read String.vi"("Name"=w287) -> ("String"=w290:string)  [unwired: 9 in, 1 out]
                n162 = Bundle("Numeric"=w289, "String"=w290) -> (→"Progress":cluster{"Numeric":dbl, "String":string})  [unwired: 1 in]
              }
              frame "" {
                n163 = property on="Progress" class="Clust (strict)"("Visible"=FALSE) -> ()  [unwired: 2 in, 2 out]
                n164 = local write "Test Name"(u16 0) -> ()
              }
            }
            n165 = property on="Test Tree" class="Tree (strict)"("Active Item Row Number"=w284, "ActiveColNum"=w284, "CellBG"=w281, "Active Item Row Number"=-1 ("Active Item:Row Number"), "CellBG"=u32 5789784 ("Color Box")) -> ()  [unwired: 2 in, 2 out]
          }
          frame "Variables" {
            w296 = string[] ["CameraPublisher", "Usage", "DB"]  # Items to initially close
            n166 = First Call?() -> (First Call?: T/F=w297:bool)
            n167 = control-ref of="Tree"() -> (w298:refnum<vi>)
            n168 = Select(t=w296, s=w297, f=string[] []) -> (s? t:f=w294:string[])
            n169 = call <vilib>:"NT Read and Format Entries as Tree.vi"("Tags to  Close"=w294, "Tree Refnum"=w298) -> ()  [unwired: 8 in, 2 out]
          }
          frame "Commands" {
            w307 = u32 5789784 ("Color Box")
            w308 = T26 {"Row"=-1, "Column"=-2} ("Active Cell:Active Cell")
            w310 = T26 {"Row"=-2, "Column"=-2} ("Active Cell:Active Cell")
            n170 = Index Array(array=w311, index=w305) -> (element=w309:u32)
            n171 = Index Array(array=w306, index=w305) -> (element=w304:T25)
            n172 = Unbundle(w304) -> ("Operation"=w303:enum16{"Update", "Clear"})  [unwired: 1 out]
            n173 = local read "Command Selection"() -> (w302:i32)
            n174 = property on="Command Selection" class="MCListbox (strict)"("ActiveCell"=w310, "CellBG"=w309, "ActiveCell"=w308, "CellBG"=w307) -> ()  [unwired: 2 in, 2 out]
            n175 = call <vilib>:"WPI_DashboardUpdate RPC Info.vi"("Operation"=w303) -> ("update"=w301:bool, "commands"=w300:string[][])  [unwired: 9 in]
            n176 = property on="Command Selection" class="MCListbox (strict)"("ItemNames"=w300) -> ()  [unwired: 2 in, 2 out]
            n177 = property on="Command Params" class="Tbl (strict)"("Active Cell"=w310, "Cell BG Color"=w309, "Active Cell"=w308, "Cell BG Color"=w307) -> ()  [unwired: 2 in, 2 out]
            n178 = call <vilib>:"WPI_DashboardUpdate Command Params.vi"("Update"=w301, "NewVal"=w302, "Commands"=w300, "Param Tbl"=w299) -> ()  [unwired: 7 in, 1 out]
          }
        }
        n179 = call <vilib>:"Connextion Info.vi"() -> ("Connected"=→"NT Connection":bool)  [unwired: 10 in, 1 out]
      }
      event "Test Tree": Value Change {
        # "Show appropriate\ncontrols"
        n180 = event-data() -> ("CtlRef"=w316:refnum<vi>, "NewVal"=w314:string)  [unwired: 1 in]
        n181 = call <vilib>:"WPI_UtilitiesGetTreeIOName.vi"("NewVal"=w314, "TreeControl in"=w316) -> ("I/O Name"=w317:string)  [unwired: 9 in]
        n182 = case shown="\"Camera\"" w317 {
          selector: w317 -> [_ w324 _ w346 w355 _]
          tunnel: w314 -> [_ _ w343 w345 _ w362]
          tunnel: cluster{string[]}[] [{["640x480", "320x240", "160x120"]}, {["Auto", "Fixed indoor", "Fixed outdoor 1", "Fixed outdoor 2", "Fixed fluorescent 1", "Fixed fluorescent 2", "Hold current"]}, {["Auto", "Flicker-free 50 Hz", "Flicker-free 60 Hz", "Hold current"]}, {["None", "Prioritize frame rate", "Prioritize image quality"]}, {["Monochrome", "Color"]}] -> [_ _ _ _ _ w361]
          frame Default {
            w319 = FALSE ("Visible")
            w318 = FALSE ("Visible")
            n183 = property on="Motor" class="Clust (strict)"("Visible"=w318) -> ()  [unwired: 2 in, 2 out]
            n184 = property on="Test Ring" class="Ring (strict)"("Visible"=w318) -> ()  [unwired: 2 in, 2 out]
            n185 = property on="Rev/Fwd" class="Clust (strict)"("Visible"=w319) -> ()  [unwired: 2 in, 2 out]
            n186 = property on="On/Off" class="Bool (strict)"("Visible"=w319) -> ()  [unwired: 2 in, 2 out]
            n187 = property on="Test Slider" class="Slide (strict)"("Visible"=w319) -> ()  [unwired: 2 in, 2 out]
          }
          frame "Analog Out", "Motor", "PWM" {
            w325 = FALSE ("Visible")
            n188 = case shown="\"Analog Out\"" w324 {
              tunnel: [1.0 ("Value") -1.0 ("Value") 0.0 ("Value")] -> w323
              tunnel: [255.0 ("Value") 1.0 ("Value") 5.0 ("Value")] -> w322
              tunnel: [128.0 ("Value") 0.0 ("Value") 0.0 ("Value")] -> w321
              tunnel: [64.0 ("Value") 0.5 ("Value") 1.0 ("Value")] -> w320
              frame "PWM" {
              }
              frame "Motor", Default {
              }
              frame "Analog Out" {
              }
            }
            n189 = property on="Motor" class="Clust (strict)"("Visible"=TRUE) -> ()  [unwired: 2 in, 2 out]
            n190 = property on="Value" class="Slide (strict)"("Value"=w321, "Scale.Minimum"=w323, "Scale.Maximum"=w322, "Scale.Increment"=w320) -> ()  [unwired: 2 in, 2 out]
            n191 = property on="On/Off" class="Bool (strict)"("Visible"=w325) -> ()  [unwired: 2 in, 2 out]
            n192 = property on="Test Slider" class="Slide (strict)"("Visible"=w325) -> ()  [unwired: 2 in, 2 out]
            n193 = property on="Test Ring" class="Ring (strict)"("Visible"=w325) -> ()  [unwired: 2 in, 2 out]
            n194 = property on="Rev/Fwd" class="Clust (strict)"("Visible"=w325) -> ()  [unwired: 2 in, 2 out]
          }
          frame "Servo" {
            w341 = FALSE ("Visible")
            n195 = call <vilib>:"NT Read Number.vi"("Name"=w343) -> ("Numeric"=w342:dbl)  [unwired: 9 in, 1 out]
            n196 = property on="Test Slider" class="Slide (strict)"("Visible"=TRUE, "Scale.Maximum"=170.0 ("Scale.Range:Maximum")) -> ()  [unwired: 2 in, 2 out]
            n197 = local write "Test Slider"(w342) -> ()
            n198 = property on="Motor" class="Clust (strict)"("Visible"=w341) -> ()  [unwired: 2 in, 2 out]
            n199 = property on="Rev/Fwd" class="Clust (strict)"("Visible"=w341) -> ()  [unwired: 2 in, 2 out]
            n200 = property on="On/Off" class="Bool (strict)"("Visible"=w341) -> ()  [unwired: 2 in, 2 out]
            n201 = property on="Test Ring" class="Ring (strict)"("Visible"=w341) -> ()  [unwired: 2 in, 2 out]
          }
          frame "Relay", "Solenoid" {
            w344 = FALSE ("Visible")
            n202 = property on="Motor" class="Clust (strict)"("Visible"=w344) -> ()  [unwired: 2 in, 2 out]
            n203 = property on="Test Slider" class="Slide (strict)"("Visible"=w344) -> ()  [unwired: 2 in, 2 out]
            n204 = Search and Replace String(input string=w345, search string="/Value  **", replace string="/Direction") -> (result string=w351:string)  [unwired: 5 in, 3 out]
            n205 = property on="Test Ring" class="Ring (strict)"("Visible"=w344) -> ()  [unwired: 2 in, 2 out]
            n206 = call <vilib>:"NT Read String.vi"("Name"=w351) -> ("String"=w349:string)  [unwired: 9 in, 1 out]
            n207 = Equal?(x="Both directions", y=w349) -> (x = y?=w347:bool)
            n208 = Not(x=w347) -> (.not. x?=w348:bool)
            n209 = property on="Rev/Fwd" class="Clust (strict)"("Visible"=w347) -> ()  [unwired: 2 in, 2 out]
            n210 = property on="On/Off" class="Bool (strict)"("Visible"=w348, "Caption.Text"=w346) -> ()  [unwired: 2 in, 2 out]
          }
          frame "Compressor", "Digital Out" {
            w354 = FALSE ("Visible")
            # "Get direction and finish"
            n211 = property on="Motor" class="Clust (strict)"("Visible"=w354) -> ()  [unwired: 2 in, 2 out]
            n212 = property on="Test Slider" class="Slide (strict)"("Visible"=w354) -> ()  [unwired: 2 in, 2 out]
            n213 = property on="Test Ring" class="Ring (strict)"("Visible"=w354) -> ()  [unwired: 2 in, 2 out]
            n214 = property on="On/Off" class="Bool (strict)"("Visible"=TRUE, "Caption.Text"=w355) -> ()  [unwired: 2 in, 2 out]
            n215 = property on="Rev/Fwd" class="Clust (strict)"("Visible"=FALSE) -> ()  [unwired: 2 in, 2 out]
          }
          frame "Camera" {
            n216 = call <vilib>:"Get Last Path Segment.vi"("String in"=w362) -> ("String out"=w363:string)  [unwired: 10 in]
            n217 = property on="On/Off" class="Bool (strict)"("Visible"=FALSE) -> ()  [unwired: 2 in, 2 out]
            n218 = property on="Motor" class="Clust (strict)"("Visible"=FALSE) -> ()  [unwired: 2 in, 2 out]
            n219 = property on="Rev/Fwd" class="Clust (strict)"("Visible"=FALSE) -> ()  [unwired: 2 in, 2 out]
            n220 = case shown="\"White Balance  **\"" w363 {
              tunnel: w362 -> [w369 w378 w387 w396 w405 _ w411]
              tunnel: w361 -> [w367 w375 w384 w393 w402 _ _]
              frame "Size  **" {
                n221 = Index Array(array=w367) -> (element=w366:cluster{string[]})  [unwired: 1 in]
                n222 = call <vilib>:"NT Read String.vi"("Name"=w369) -> ("String"=w368:string)  [unwired: 9 in, 1 out]
                n223 = Unbundle(w366) -> (w364:string[])
                n224 = Match First String(2:w364, 3:w368) -> (0:w365:i32)  [unwired: 1 out]
                n225 = property on="Test Ring" class="Ring (strict)"("Value"=w365, "Strings []"=w364) -> ()  [unwired: 2 in, 2 out]
                n226 = property on="Test Ring" class="Ring (strict)"("Visible"=TRUE) -> ()  [unwired: 2 in, 2 out]
                n227 = property on="Test Slider" class="Slide (strict)"("Visible"=FALSE) -> ()  [unwired: 2 in, 2 out]
              }
              frame "White Balance  **" {
                n228 = Index Array(array=w375, index=1) -> (element=w376:cluster{string[]})
                n229 = call <vilib>:"NT Read String.vi"("Name"=w378) -> ("String"=w377:string)  [unwired: 9 in, 1 out]
                n230 = Unbundle(w376) -> (w373:string[])
                n231 = Match First String(2:w373, 3:w377) -> (0:w372:i32)  [unwired: 1 out]
                n232 = property on="Test Ring" class="Ring (strict)"("Value"=w372, "Strings []"=w373) -> ()  [unwired: 2 in, 2 out]
                n233 = property on="Test Ring" class="Ring (strict)"("Visible"=TRUE) -> ()  [unwired: 2 in, 2 out]
                n234 = property on="Test Slider" class="Slide (strict)"("Visible"=FALSE) -> ()  [unwired: 2 in, 2 out]
              }
              frame "Exposure  **" {
                n235 = Index Array(array=w384, index=2) -> (element=w385:cluster{string[]})
                n236 = call <vilib>:"NT Read String.vi"("Name"=w387) -> ("String"=w386:string)  [unwired: 9 in, 1 out]
                n237 = Unbundle(w385) -> (w381:string[])
                n238 = Match First String(2:w381, 3:w386) -> (0:w382:i32)  [unwired: 1 out]
                n239 = property on="Test Ring" class="Ring (strict)"("Value"=w382, "Strings []"=w381) -> ()  [unwired: 2 in, 2 out]
                n240 = property on="Test Ring" class="Ring (strict)"("Visible"=TRUE) -> ()  [unwired: 2 in, 2 out]
                n241 = property on="Test Slider" class="Slide (strict)"("Visible"=FALSE) -> ()  [unwired: 2 in, 2 out]
              }
              frame "Exposure Priority  **" {
                n242 = Index Array(array=w393, index=3) -> (element=w394:cluster{string[]})
                n243 = call <vilib>:"NT Read String.vi"("Name"=w396) -> ("String"=w395:string)  [unwired: 9 in, 1 out]
                n244 = Unbundle(w394) -> (w390:string[])
                n245 = Match First String(2:w390, 3:w395) -> (0:w391:i32)  [unwired: 1 out]
                n246 = property on="Test Ring" class="Ring (strict)"("Value"=w391, "Strings []"=w390) -> ()  [unwired: 2 in, 2 out]
                n247 = property on="Test Ring" class="Ring (strict)"("Visible"=TRUE) -> ()  [unwired: 2 in, 2 out]
                n248 = property on="Test Slider" class="Slide (strict)"("Visible"=FALSE) -> ()  [unwired: 2 in, 2 out]
              }
              frame "Color Enable  **" {
                n249 = Index Array(array=w402, index=4) -> (element=w403:cluster{string[]})
                n250 = call <vilib>:"NT Read String.vi"("Name"=w405) -> ("String"=w404:string)  [unwired: 9 in, 1 out]
                n251 = Unbundle(w403) -> (w399:string[])
                n252 = Match First String(2:w399, 3:w404) -> (0:w400:i32)  [unwired: 1 out]
                n253 = property on="Test Ring" class="Ring (strict)"("Value"=w400, "Strings []"=w399) -> ()  [unwired: 2 in, 2 out]
                n254 = property on="Test Ring" class="Ring (strict)"("Visible"=TRUE) -> ()  [unwired: 2 in, 2 out]
                n255 = property on="Test Slider" class="Slide (strict)"("Visible"=FALSE) -> ()  [unwired: 2 in, 2 out]
              }
              frame Default {
                n256 = property on="Test Ring" class="Ring (strict)"("Visible"=FALSE) -> ()  [unwired: 2 in, 2 out]
                n257 = property on="Test Slider" class="Slide (strict)"("Visible"=FALSE) -> ()  [unwired: 2 in, 2 out]
              }
              frame "Brightness  **", "Color Level  **", "Compression  **", "FPS  **", "Sharpness  **" {
                n258 = call <vilib>:"NT Read Number.vi"("Name"=w411) -> ("Numeric"=w410:dbl)  [unwired: 9 in, 1 out]
                n259 = local write "Test Slider"(w410) -> ()
                n260 = property on="Test Slider" class="Slide (strict)"("Visible"=TRUE, "Scale.Maximum"=100.0 ("Scale.Range:Maximum")) -> ()  [unwired: 2 in, 2 out]
                n261 = property on="Test Ring" class="Ring (strict)"("Visible"=FALSE) -> ()  [unwired: 2 in, 2 out]
              }
            }
          }
        }
        n262 = property on="Progress" class="Clust (strict)"("Visible"=FALSE) -> ()  [unwired: 2 in, 2 out]
      }
      event "Test Name": Mouse Enter {
        # "Populate the ring with the list of tests"
        n263 = event-data() -> ()  [unwired: 1 in, 1 out]
        n264 = call <vilib>:"NT Read String Array.vi"("Name"="TestMode/TestList") -> ("String Array"=w419:string[])  [unwired: 9 in, 1 out]
        n265 = Build Array (concatenate)("Select the test to run...", w419) -> (w418:string[])
        n266 = property on="Test Name" class="Ring (strict)"("Strings []"=w418) -> ()  [unwired: 2 in, 2 out]
      }
      event "Test Name": Value Change {
        w421 = FALSE ("Visible")
        # "Tell the robot the test name to run"
        n267 = event-data() -> ("NewVal"=w425:u16)  [unwired: 1 in]
        n268 = property on="Test Name" class="Ring (strict)"() -> ("Strings []"=w426:string[])  [unwired: 2 in, 2 out]
        n269 = local write "Progress"(T6 {"Test Progress"=0, "Test Progress Text"=""} ("Progress")) -> ()
        n270 = Index Array(array=w426, index=w425) -> (element=w424:string)
        n271 = call <vilib>:"NT Write String.vi"("String"=w424, "Name"="TestMode/TestName") -> ()  [unwired: 9 in, 1 out]
        n272 = property on="Progress" class="Clust (strict)"("Visible"=TRUE) -> ()  [unwired: 2 in, 2 out]
        n273 = property on="Motor" class="Clust (strict)"("Visible"=w421) -> ()  [unwired: 2 in, 2 out]
        n274 = property on="Test Slider" class="Slide (strict)"("Visible"=w421) -> ()  [unwired: 2 in, 2 out]
        n275 = property on="On/Off" class="Bool (strict)"("Visible"=w421) -> ()  [unwired: 2 in, 2 out]
        n276 = property on="Rev/Fwd" class="Clust (strict)"("Visible"=w421) -> ()  [unwired: 2 in, 2 out]
        n277 = property on="Test Ring" class="Ring (strict)"("Visible"=w421) -> ()  [unwired: 2 in, 2 out]
      }
      event "Select Auto": Mouse Enter {
        # "Populate the combo box with the list of autonomous options"
        n278 = event-data() -> ()  [unwired: 1 in, 1 out]
        n279 = call <vilib>:"NT Read String Array.vi"("Name"="Auto List") -> ("String Array"=w428:string[])  [unwired: 9 in, 1 out]
        n280 = property on="Select Auto" class="CmbBox"("Strings[]"=w428) -> ()  [unwired: 2 in, 2 out]
      }
      event "Select Auto": Value Change {
        # "User modified the Auto Selection. Write to NT variable so robot knows."
        n281 = event-data() -> ("NewVal"=w431:string)  [unwired: 1 in]
        n282 = call <vilib>:"NT Write String.vi"("String"=w431, "Name"="Auto Selector") -> ()  [unwired: 9 in, 1 out]
      }
      event "Command Selection": Value Change {
        # "Get the params and show in table"
        n283 = event-data() -> ("NewVal"=w437:i32)  [unwired: 1 in]
        n284 = property on="Command Selection" class="MCListbox (strict)"() -> ("ItemNames"=w435:string[][])  [unwired: 2 in, 2 out]
        n285 = call <vilib>:"WPI_DashboardUpdate Command Params.vi"("NewVal"=w437, "Commands"=w435, "Param Tbl"=w436) -> ()  [unwired: 8 in, 1 out]
      }
      event "Execute Command": Value Change {
        # "Started one, Unique ID holds\nresponse"
        n286 = event-data() -> ()  [unwired: 1 in, 1 out]
        n287 = property on="Command Selection" class="MCListbox (strict)"() -> ("ItemNames"=w448:string[][])  [unwired: 2 in, 2 out]
        n288 = Index Array(array=w448, index (row)="Command Selection", index (col)=0) -> (element=w446:string)
        n289 = call <vilib>:"Invoke Commands.vi"("Command Params"="Command Params", "Function Name"=w446) -> ("Params"=w442:u8, "Started"=w441:bool)  [unwired: 7 in, 1 out]
        n290 = Array Subset(array="Command Params", length (row)=w442) -> (w443:string[][])  [unwired: 3 in]
        n291 = Select(t="Executing" ("Cmd Status"), s=w441, f="" ("Cmd Status")) -> (s? t:f=→"Cmd Status":string)
      }
      event "Command Selection": Double Click {
        n292 = event-data() -> ("Row"=w456:i32)  [unwired: 1 in]
        n293 = property on="Command Selection" class="MCListbox (strict)"() -> ("ItemNames"=w459:string[][])  [unwired: 2 in, 2 out]
        n294 = local read "Command Params"() -> (w455:string[][])
        n295 = Index Array(array=w459, index (row)=w456, index (col)=0) -> (element=w457:string)
        n296 = call <vilib>:"Invoke Commands.vi"("Command Params"=w455, "Function Name"=w457) -> ("Params"=w454:u8, "Started"=w449:bool)  [unwired: 7 in, 1 out]
        n297 = Array Subset(array=w455, length (row)=w454) -> (w453:string[][])  [unwired: 3 in]
        n298 = Select(t="Executing" ("Cmd Status"), s=w449, f="" ("Cmd Status")) -> (s? t:f=w450:string)
        n299 = local write "Cmd Status"(w450) -> ()
      }
      event "CheckList": Double Click {
        # "Shift clears all"
        # "Update symbols on the listbox"
        n300 = event-data() -> ("PlatMods.Shift"=w461:bool, "Row"=w463:i32)  [unwired: 1 in]
        n301 = case shown="True" w461 {
          tunnel: w463 -> [w467 _]
          tunnel: 1 -> [w466 _]
          frame False {
            n302 = property on="CheckList" class="LstBox (strict)"() -> ("Item Symbols"=w465:i32[])  [unwired: 2 in, 2 out]
            n303 = Replace Array Subset(array=w465, new element=w466, index=w467) -> (w464:i32[])
            n304 = property on="CheckList" class="LstBox (strict)"("Item Symbols"=w464) -> ()  [unwired: 2 in, 2 out]
          }
          frame True {
            w468 = 0 ("Top Row")
            n305 = property on="CheckList" class="LstBox (strict)"() -> ("Number of Rows"=w470:u32)  [unwired: 2 in, 2 out]
            n306 = Initialize Array(0, w470) -> (w469:i32[])
            n307 = property on="CheckList" class="LstBox (strict)"("Top Row"=w468, "Value"=w468, "Item Symbols"=w469) -> ()  [unwired: 2 in, 2 out]
          }
        }
      }
      event "CheckList": Key Down {
        # "Update symbols on the listbox\nLeft and right keys check and uncheck"
        n308 = event-data() -> ("VKey"=w474:T23)  [unwired: 1 in]
        n309 = case shown="\"Left\", \"Right\"" w474 {
          selector: w474 -> [w479 _]
          tunnel: eventvkey."Left" ("VKey") -> [w477 _]
          frame "Left", "Right" {
            n310 = Equal?(x=w477, y=w479) -> (x = y?=w478:bool)
            n311 = Select(t=0, s=w478, f=1) -> (s? t:f=w480:i32)
            n312 = property on="CheckList" class="LstBox (strict)"() -> ("Item Symbols"=w483:i32[])  [unwired: 2 in, 2 out]
            n313 = Replace Array Subset(array=w483, new element=w480, index="CheckList") -> (w482:i32[])
            n314 = property on="CheckList" class="LstBox (strict)"("Item Symbols"=w482) -> ()  [unwired: 2 in, 2 out]
          }
          frame Default {
          }
        }
      }
      event "Motor.Enable": Value Change {
        # "When the test mode otor enable helper is set, update that\ntree row item's value"
        n315 = event-data() -> ("NewVal"=w489:bool)  [unwired: 1 in]
        n316 = Unbundle("Motor") -> ("Value"=w488:dbl)  [unwired: 1 out]
        n317 = Select(t=w488, s=w489, f=0.0) -> (s? t:f=w486:dbl)
        n318 = call <vilib>:"NT Write Number.vi"("Numeric"=w486, "Name"=w485) -> ()  [unwired: 9 in, 1 out]
      }
      event "Test Slider": Value Change {
        # "When the test mode slider helper is set, update that\ntree row item's value"
        n319 = event-data() -> ("NewVal"=w492:dbl)  [unwired: 1 in]
        n320 = call <vilib>:"NT Write Number.vi"("Numeric"=w492, "Name"=w493) -> ()  [unwired: 9 in, 1 out]
      }
      event "On/Off": Value Change {
        # "When the test mode on/off helper value is set, update that\ntree row item's value"
        n321 = event-data() -> ("NewVal"=w497:bool)  [unwired: 1 in]
        n322 = Boolean To (0,1)(Boolean=w497) -> (0, 1=w496:i16)
        n323 = call <vilib>:"NT Write Number.vi"("Numeric"=w496, "Name"=w495) -> ()  [unwired: 9 in, 1 out]
      }
      event "Rev/Fwd": Value Change {
        # "When the test mode helper value for relays is set, update that\ntree row item's value"
        n324 = event-data() -> ("NewVal.Forward"=w505:bool, "NewVal.Reverse"=w504:bool)  [unwired: 1 in]
        n325 = Boolean To (0,1)(Boolean=w505) -> (0, 1=w501:i16)
        n326 = Boolean To (0,1)(Boolean=w504) -> (0, 1=w503:i16)
        n327 = Negate(x=w503) -> (-x=w502:i16)
        n328 = Add(x=w501, y=w502) -> (x+y=w500:i16)
        n329 = call <vilib>:"NT Write Number.vi"("Numeric"=w500, "Name"=w499) -> ()  [unwired: 9 in, 1 out]
      }
      event "Test Ring": Value Change {
        # "When a test mode helper value is selected from the ring,\nset the tree item's variable to the string value"
        n330 = event-data() -> ("NewVal"=w509:u16)  [unwired: 1 in]
        n331 = property on="Test Ring" class="Ring (strict)"() -> ("Strings []"=w510:string[])  [unwired: 2 in, 2 out]
        n332 = Index Array(array=w510, index=w509) -> (element=w508:string)
        n333 = call <vilib>:"NT Write String.vi"("String"=w508, "Name"=w507) -> ()  [unwired: 9 in, 1 out]
      }
      event "Rec Mode": Value Change {
        # "Update globals for recording mode and path to read log from.\nClear when logging and let NetworkTables set path for vision to\nuse."
        n334 = event-data() -> ("NewVal"=w521:enum32{"Stop", "Record", "Playback"})  [unwired: 1 in]
        n335 = global write "WPI_DashboardLogging Global.vi" "Logging Filename"(path "") -> ()
        n336 = global write "WPI_DashboardLogging Global.vi" "Recording"(w521) -> ()
        n337 = case shown="\"Playback\"" w521 {
          tunnel: w520 -> [_ w523 w532]
          tunnel: [_ _ w531] -> w518
          tunnel: [_ _ w530] -> _
          tunnel: w516 -> [_ _ w528]
          tunnel: cluster{i32, i32} {-250, 170} -> [_ _ w527]
          tunnel: [_ _ T24 {"Image Size"=TRUE, "Image Type"=TRUE, "Pixel Value"=TRUE, "ROI Information"=TRUE, "Zoom Factor"=FALSE} ("Image Information Shown:All Elements")] -> w511
          tunnel: [_ _ TRUE ("Zoom Factor")] -> w512
          tunnel: w514 -> [_ _ w524]
          frame Default {
          }
          frame "Stop", "Record" {
            # "Place Window too"
            n338 = invoke class="VI" method="FP.Close"(reference=w523) -> (reference out=w522:refnum<vi>)  [unwired: 2 in, 2 out]
            n339 = invoke class="VI" method="Abort VI"(reference=w522) -> ()  [unwired: 2 in, 3 out]
          }
          frame "Playback" {
            n340 = call "Open Playback Panel.vi"("Offset"=w527, "DB VI Ref"=w528, "Playback in"=w532) -> ("Playback out"=w529:refnum<vi>)  [unwired: 8 in]
            n341 = register-events(w529, w524) -> (reference out=w531:refnum<event-registration>, error out=w530:errorcluster)  [unwired: 2 in]
          }
        }
        n342 = property on="Camera Image Right" class="ImageControl"("Image Information Shown"=w511, "Image Information Visible"=w512) -> ()  [unwired: 2 in, 2 out]
        n343 = property on="Camera Image" class="ImageControl"("Image Information Shown"=w511, "Image Information Visible"=w512) -> ()  [unwired: 2 in, 2 out]
        n344 = call <vilib>:"WPI_DashboardNT Log FieldName Cache.vi"("Operation"=enum16{"Lookup/Add", "Index", "Clear"}."Clear") -> ()  [unwired: 8 in, 3 out]
      }
      event Panel Close {
        w534 = enum32{"Stop", "Record", "Playback"}."Stop" ("Rec Mode")
        # "Playback window has been closed, abort"
        n345 = event-data() -> ()  [unwired: 1 in, 4 out]
        n346 = local write "Rec Mode"(w534) -> ()
        n347 = global write "WPI_DashboardLogging Global.vi" "Recording"(w534) -> ()
      }
      event Panel Close {
        # "Abort playback window and ourself"
        n348 = event-data() -> ()  [unwired: 1 in, 4 out]
        n349 = invoke class="VI" method="FP.Close"(reference=w538) -> (reference out=w537:refnum<vi>)  [unwired: 2 in, 2 out]
        n350 = invoke class="VI" method="Abort VI"(reference=w537) -> (error out=w536:errorcluster)  [unwired: 2 in, 2 out]
        n351 = invoke class="VI" method="Abort VI"(error in=w536) -> ()  [unwired: 2 in, 3 out]
      }
      event User Event {
        n352 = event-data() -> ("IDs"=w545:cluster{"RPC field ID":u16, "Unique ID":u16}, "String"=w544:string)  [unwired: 1 in]
        n353 = Bundle("IDs"=w545, "String"=w544) -> (w543:T10)  [unwired: 1 in]
        n354 = call <vilib>:"Retrieve RPC Response.vi"("RPC Response"=w543) -> ("Output"=w541:string[][])  [unwired: 10 in]
        n355 = Build Array (concatenate)(w539, w541) -> (w540:string[][])
        n356 = local write "Command Params"(w540) -> ()
        n357 = local write "Cmd Status"("" ("Cmd Status")) -> ()
      }
      event "Tree": Double Click {
        n358 = event-data() -> ("PlatMods"=w551:T27, "Tag"=w548:string)  [unwired: 1 in]
        n359 = Unbundle(w551) -> ("Shift"=w550:bool)  [unwired: 4 out]
        n360 = String Subset(string=w548, length (rest)=1 ("length (rest)")) -> (substring=w547:string)  [unwired: 1 in]
        n361 = Not(x=w550) -> (.not. x?=w549:bool)
        n362 = case shown="\"/\"" w547 {
          tunnel: w548 -> [_ w554]
          tunnel: w549 -> [_ w553]
          frame Default {
          }
          frame "/" {
            n363 = call <vilib>:"NT Update Persistence.vi"("Persistence"=w553, "Name"=w554) -> ()  [unwired: 9 in, 1 out]
          }
        }
      }
    }
  }
  n364 = while {
    tunnel: w76 -> [w556]
    i -> [w559]
    stop <- FALSE stop-if-true
    n365 = Wait (ms)(milliseconds to wait=u32 100) -> ()  [unwired: 1 out]
    n366 = case shown="\"Stop\", Default" "Rec Mode" {
      tunnel: w559 -> [_ _ w574]
      tunnel: [u32 2829099 ("Base Color") u32 11141120 ("Target Color") w563] -> w555
      frame "Stop", Default {
        # "Reset the color, extra updates don't cost much"
      }
      frame "Record" {
      }
      frame "Playback" {
        # "Playback"
        n367 = Quotient & Remainder(x=w574, y=u32 50 ("milliseconds to wait")) -> (x-y*floor(x/y)=w570:u32)  [unwired: 1 out]
        n368 = Divide(x=w570, y=u32 50 ("milliseconds to wait")) -> (x/y=w567:dbl)
        n369 = Multiply(x=6.283185307179586, y=w567) -> (x*y=w572:dbl)
        n370 = Sine(x=w572) -> (sin(x)=w571:dbl)
        n371 = Absolute Value(x=w571) -> (abs(x)=w564:dbl)
        n372 = call "Interpolate RGB Color.vi"("Proportion"=w564, "Target Color"=u32 30976, "Base Color"=u32 2829099) -> ("Result Color"=w563:u32)  [unwired: 8 in]
      }
    }
    n373 = property class="Pane"(reference=w556, "PaneColor"=w555) -> ()  [unwired: 1 in, 2 out]
  }
  n374 = local write "Dashboard Tab"(T8."Drive" ("Dashboard Tab")) -> ()
  n375 = property on="On/Off" class="Bool (strict)"("Visible"=w47) -> ()  [unwired: 2 in, 2 out]
  n376 = property on="Motor" class="Clust (strict)"("Visible"=w47) -> ()  [unwired: 2 in, 2 out]
  n377 = property on="Progress" class="Clust (strict)"("Visible"=w47) -> ()  [unwired: 2 in, 2 out]
  n378 = property on="Test Ring" class="Ring (strict)"("Visible"=w47) -> ()  [unwired: 2 in, 2 out]
  n379 = property on="Rev/Fwd" class="Clust (strict)"("Visible"=w47) -> ()  [unwired: 2 in, 2 out]
  n380 = while {
    tunnel: u16 1741 ("timeout ms (25000)") -> [w576]
    stop <- FALSE stop-if-true
    n381 = TCP Create Listener(10:w576) -> (0:w575:errorcluster, 3:w577:refnum<k5>)  [unwired: 4 in, 1 out]
    n382 = case shown="Error" w575 {
      selector: w575 -> [w579 _]
      tunnel: w577 -> [w580 _]
      frame No Error {
        n383 = while {
          tunnel: w580 -> [w583]
          tunnel: w579 -> [w582]
          stop <- FALSE stop-if-true
          n384 = TCP Wait On Listener(8:w582, 11:w583) -> (0:w584:errorcluster, 4:w585:refnum<k5>)  [unwired: 2 in, 3 out]
          n385 = local write "TCP"(w585) -> ()
          n386 = case shown="No Error" w584 {
            frame No Error {
            }
            frame Error {
              n387 = Wait (ms)(milliseconds to wait=u32 1000) -> ()  [unwired: 1 out]
            }
          }
        }
      }
      frame Error {
        n388 = Wait (ms)(milliseconds to wait=u32 1000) -> ()  [unwired: 1 out]
      }
    }
  }
  n389 = local write "Command Selection"(u16 0 ("milliseconds to wait")) -> ()
  n390 = local write "Command Params"(string[][] [] ("Command Params")) -> ()
  n391 = global write "WPI_DashboardLogging Global.vi" "Recording"(w70) -> ()
  n392 = local write "Rec Mode"(w70) -> ()
  n393 = call <vilib>:"NT Write String.vi"("String"="Select Auto", "Name"="Auto Selector") -> ()  [unwired: 9 in, 1 out]
  n394 = property on="Drive" class="TabCtl (strict)"() -> ("Pages"=w2:refnum<vi>[])  [unwired: 2 in, 2 out]
  n395 = call-poly <vilib>:"Read Delimited Spreadsheet.vi"("file path (dialog if empty)"=path "C:/Users/bhanu/Desktop/DriveCalsTest.csv", "transpose? (F)"=TRUE, "delimiter (\\t)"="," ("delimiter (\\t)")) -> ("all rows"=w9:string[][])  [unwired: 7 in, 5 out]
  n396 = Index Array(array=w9, index (col) #1=0 ("disabled index (col)")) -> (element #1=w8:string[], element #2=w6:string[])  [unwired: 3 in]
  n397 = Index Array(array=w2, index #1=0 ("index")) -> (element #1=w4:refnum<vi>)  [unwired: 4 in, 4 out]
  n398 = property class="Page"(reference=w4) -> ("ControlsOnPage"=w1:refnum<vi>[])  [unwired: 1 in, 2 out]
  n399 = disable-structure shown="Disabled" {
    frame Disabled {
      n400 = property on="Drive" class="TabCtl (strict)"() -> ("Pages"=w588:refnum<vi>[])  [unwired: 2 in, 2 out]
      n401 = Index Array(array=w588, index #1=0 ("index")) -> (element #1=w598:refnum<vi>)  [unwired: 4 in, 4 out]
      n402 = property class="Page"(reference=w598) -> ("ControlsOnPage"=w596:refnum<vi>[])  [unwired: 1 in, 2 out]
      n403 = Read from Text File(file (use dialog)=path "C:/Users/bhanu/Desktop/DriveCalsTest.csv" ("file path (dialog if empty)"), count=-1) -> (text=w593:string)  [unwired: 2 in, 3 out]
      n404 = Spreadsheet String To Array(delimiter (Tab)=",", format string="%f", spreadsheet string=w593, array type (2D Dbl)=dbl[][] []) -> (array=w589:dbl[][])
      n405 = for {
        tunnel: w596 -> [w600] mode=indexing
        tunnel: w589 -> [w599] mode=indexing
        n406 = property class="Ctl"(reference=w600, "Value"=w599) -> ()  [unwired: 1 in, 2 out]
      }
    }
    frame Enabled {
    }
  }
  n407 = for {
    tunnel: w8 -> [w605]
    tunnel: w6 -> [w602]
    tunnel: w1 -> [w601] mode=indexing
    n408 = property class="Ctl"(reference=w601) -> (reference out=w607:refnum<vi>, "Label.Text"=w609:string)  [unwired: 1 in, 1 out]
    n409 = Search 1D Array(1D array=w605, element=w609, start index (0)=0) -> (index of element=w604:i32)
    n410 = Greater Or Equal To 0?(x=w604) -> (x >= 0?=w606:bool)
    n411 = Index Array(array=w602, index=w604) -> (element=w603:string)
    n412 = case shown="True" w606 {
      tunnel: w607 -> [_ w612]
      tunnel: w603 -> [_ w610]
      frame False {
      }
      frame True {
        n413 = Fract/Exp String To Number(string=w610) -> (number=w611:dbl)  [unwired: 3 in, 1 out]
        n414 = property class="Ctl"(reference=w612, "Value"=w611) -> ()  [unwired: 1 in, 2 out]
      }
    }
  }
  n415 = disable-structure shown="Disabled" {
    frame Disabled {
      n416 = call-poly <vilib>:"NT Read Value.vi"("Name"="IntakeCals") -> ("String"=w624:string)  [unwired: 9 in, 1 out]
      n417 = call-poly <vilib>:"NT Read Value.vi"("Name"="AutoTargetCals") -> ("String"=w617:string)  [unwired: 9 in, 1 out]
      n418 = call-poly <vilib>:"NT Read Value.vi"("Name"="TurretCals") -> ("String"=w634:string)  [unwired: 9 in, 1 out]
      n419 = call-poly <vilib>:"NT Read Value.vi"("Name"="ClimbCals") -> ("String"=w641:string)  [unwired: 9 in, 1 out]
      n420 = call-poly <vilib>:"NT Read Value.vi"("Name"="DriveCals") -> ("String"=w662:string)  [unwired: 9 in, 1 out]
      n421 = Spreadsheet String To Array(format string="%f", spreadsheet string=w624, array type (2D Dbl)=dbl[] []) -> (array=w623:dbl[])  [unwired: 1 in]
      n422 = Spreadsheet String To Array(format string="%f", spreadsheet string=w617, array type (2D Dbl)=dbl[] []) -> (array=w616:dbl[])  [unwired: 1 in]
      n423 = Spreadsheet String To Array(format string="%f", spreadsheet string=w634, array type (2D Dbl)=dbl[] []) -> (array=w633:dbl[])  [unwired: 1 in]
      n424 = Index Array(array=w623) -> (element #1=w622:dbl, element #2=w621:dbl)  [unwired: 2 in]
      n425 = Index Array(array=w616) -> (element #1=w615:dbl, element #2=w614:dbl, element #3=w613:dbl)  [unwired: 3 in]
      n426 = Spreadsheet String To Array(format string="%f", spreadsheet string=w641, array type (2D Dbl)=dbl[] []) -> (array=w644:dbl[])  [unwired: 1 in]
      n427 = Index Array(array=w633) -> (element #1=w630:dbl, element #2=w631:dbl, element #3=w632:dbl, element #4=w629:dbl, element #5=w628:dbl)  [unwired: 5 in]
      n428 = Spreadsheet String To Array(format string="%f", spreadsheet string=w662, array type (2D Dbl)=dbl[] []) -> (array=w665:dbl[])  [unwired: 1 in]
      n429 = Index Array(array=w644) -> (element #1=w640:dbl, element #2=w639:dbl, element #3=w638:dbl)  [unwired: 3 in]
      n430 = property on="Intake Speed" class="DigNum (strict)"("Value"=w621) -> ()  [unwired: 2 in, 2 out]
      n431 = property on="Top IR Threshold" class="DigNum (strict)"("Value"=w622) -> ()  [unwired: 2 in, 2 out]
      n432 = property on="Turret Upper Limit" class="DigNum (strict)"("Value"=w630) -> ()  [unwired: 2 in, 2 out]
      n433 = property on="Turret Lower Limit" class="DigNum (strict)"("Value"=w631) -> ()  [unwired: 2 in, 2 out]
      n434 = property on="Climb P" class="DigNum (strict)"("Value"=w640) -> ()  [unwired: 2 in, 2 out]
      n435 = property on="Climb I" class="DigNum (strict)"("Value"=w639) -> ()  [unwired: 2 in, 2 out]
      n436 = property on="Climb D" class="DigNum (strict)"("Value"=w638) -> ()  [unwired: 2 in, 2 out]
      n437 = Index Array(array=w665) -> (element #1=w646:dbl, element #2=w647:dbl, element #3=w648:dbl, element #4=w649:dbl, element #5=w650:dbl, element #6=w651:dbl, element #7=w652:dbl, element #8=w653:dbl, element #9=w654:dbl, element #10=w655:dbl, element #11=w656:dbl, element #12=w657:dbl, element #13=w658:dbl, element #14=w659:dbl, element #15=w660:dbl, element #16=w661:dbl)  [unwired: 16 in]
      n438 = property on="Left P" class="DigNum (strict)"("Value"=w646) -> ()  [unwired: 2 in, 2 out]
      n439 = property on="Left I" class="DigNum (strict)"("Value"=w647) -> ()  [unwired: 2 in, 2 out]
      n440 = property on="Left D" class="DigNum (strict)"("Value"=w648) -> ()  [unwired: 2 in, 2 out]
      n441 = property on="Left F" class="DigNum (strict)"("Value"=w649) -> ()  [unwired: 2 in, 2 out]
      n442 = property on="Right P" class="DigNum (strict)"("Value"=w654) -> ()  [unwired: 2 in, 2 out]
      n443 = property on="Right I" class="DigNum (strict)"("Value"=w655) -> ()  [unwired: 2 in, 2 out]
      n444 = property on="Right D" class="DigNum (strict)"("Value"=w656) -> ()  [unwired: 2 in, 2 out]
      n445 = property on="Right F" class="DigNum (strict)"("Value"=w657) -> ()  [unwired: 2 in, 2 out]
    }
    frame Enabled {
    }
  }
